vi "GUI.vi"(8 "Error In":errorcluster, 11 "Data in":T6={"Console log"="", "GUI_Events"={"To_GUI-Producer"=refnum, "To_GUI-Error_message"=refnum, "To_GUI-msg_list"=refnum, "To_GUI-Session"=refnum, "To_GUI-Pre-Session"=refnum, "To_GUI-Consumer"=refnum}, "Function_Queue"={"Queue_MIDI_Handler"=refnum, "Queue_Session"=refnum, "Queue_Producer"=refnum, "Queue_Consumer"=refnum}, "Timout-Time[ms]"=0, "MIDI-Messages"=[], "Com Session State"=enum."Active Session", "Result Data"={"Diff"=[], "Tx Byte"=[], "Rx Byte"=[], "Send Log"=[], "Parsed Data"={"Tx MIDI Tag"=[], "Tx MIDI Parsed Data"=[], "Tx Error"=[], "Tx Running States"=[], "Rx MIDI Tag"=[], "Rx MIDI Parsed Data"=[], "Rx Error"=[], "Rx Running States"=[], "Diff"=[]}}, "Get #"=[], "CPU(ms)"=0}) -> (0 "Error Out":errorcluster, 3 "Data out":T6={"Console log"="", "GUI_Events"={"To_GUI-Producer"=refnum, "To_GUI-Error_message"=refnum, "To_GUI-msg_list"=refnum, "To_GUI-Session"=refnum, "To_GUI-Pre-Session"=refnum, "To_GUI-Consumer"=refnum}, "Function_Queue"={"Queue_MIDI_Handler"=refnum, "Queue_Session"=refnum, "Queue_Producer"=refnum, "Queue_Consumer"=refnum}, "Timout-Time[ms]"=0, "MIDI-Messages"=[], "Com Session State"=enum."Active Session", "Result Data"={"Diff"=[], "Tx Byte"=[], "Rx Byte"=[], "Send Log"=[], "Parsed Data"={"Tx MIDI Tag"=[], "Tx MIDI Parsed Data"=[], "Tx Error"=[], "Tx Running States"=[], "Rx MIDI Tag"=[], "Rx MIDI Parsed Data"=[], "Rx Error"=[], "Rx Running States"=[], "Diff"=[]}}, "Get #"=[], "CPU(ms)"=0})   [LabVIEW 2019]
doc: "The main Graphical User Interface"
uses:
  Common/Controls/Application_Data.ctl
  Common/Controls/App_Events.ctl
  Common/Controls/App_Queues.ctl
  Common/Controls/Application_Message.ctl
  Common/Controls/Application_State.ctl
  MIDI/Controls/MIDI-Message_Array.ctl
  MIDI/Controls/MIDI-Message_Cluster.ctl
  MIDI/Controls/Meta_Commands.ctl
  Producer/Controls/Session_State.ctl
  Consumer/Controls/Consumer_Result.ctl
  Consumer/Controls/Parsed_Data.ctl
  Common/Controls/Communication_Protocols.ctl
  Producer/Controls/Serial Settings (Remove).ctl
  <vilib>/Utility/error.llb/DialogType.ctl
  <vilib>/Utility/miscctls.llb/LVPointTypeDef.ctl
  Common/Controls/Communication_Settings.ctl
  Producer/Controls/Prod - Tx_Info.ctl
  <vilib>/Utility/file.llb/Write Delimited Spreadsheet (string).vi
panel:
  in  "BtnG: Minimize":bool
  in  "BtnG: Stop Button":bool
  in  "GUI Tab":T1(tab)
  in  "BtnM: All":bool
  in  "Rx Protocol":T2
  in  "Tx Protocol":T2
  in  "BtnM: Import Send":bool
  in  "BtnM: Preview":bool
  in  "BtnMS: Compose Message":bool
  in  "BtnM: Clear Send":bool
  in  "List: Send":i32(listbox)
  in  "List: MIDI Messages":i32(listbox)
  in  "BtnM: Load Messages":bool
  in  "BtnM: Add to Send":bool
  in  "BtnM: Save":bool
  in  "Custom Message":T3
  in  "BtnM: Cancel/Deinitiate":bool
  in  "BtnM: Initiate Producer":bool
  in  "BtnM: Update Settings":bool
  in  "Serial Communication":T4={"Baud rate"=31250, "Tx Port"="", "Rx Port"=""}
  out "Total amount of bytes to send":i32
  out "Strings":string[](array[string])
  out "Bytesize":i32[](array[numeric])
  out "Datatype":T5[](array[typedef])
  in  "BtnS: Stop Session":bool
  in  "BtnSI: Inspect Session":bool
  in  "BtnS: Pause Session":bool
  in  "BtnS: Start/Resume Session":bool
  in  "BtnI: Inspect Parsing":bool
  out "Diff bytes":i16
  out "Bytes lost":i32
  out "Data error?":bool
  out "Get #":i32
  in  "Get #":bool[](array[boolean])
  in  "BtnI: Save Data as Textfile":bool
  in  "BtnI: Export Send":bool
  in  "Scrollbar":i32(c297)
  out "Send Log":string[](array[string])
  out "Diff":bool[](array[boolean])
  out "Rx Log":string[](array[string])
  out "Tx Log":string[](array[string])
  in  "BtnI: Back 2 Main":bool
  in  "First Rx Failure":i32
  in  "BtnI:  Add Space":bool
  in  "Where Rx should be":i32
  in  "Scrollbar Parse":i32(c297)
  out "Rx Running States":string[](array[string])
  out "Rx Error?":bool[](array[boolean])
  out "Rx MIDI Message Type":string[](array[string])
  out "Rx Parsed Data":string[](array[string])
  out "Diff":bool[](array[boolean])
  out "Tx Error?":bool[](array[boolean])
  out "Tx Running States":string[](array[string])
  out "Tx Parsed Data":string[](array[string])
  out "Tx MIDI Message Type":string[](array[string])
  in  "BtnI: Back 2 Main 2":bool
  out "GUI Console log":string
  out "Error Message":string
  out "Error Loop":string
  out "VI Path":path
  out "VI-filename":string
  out "Revision Number":u32
  out "VI-Name":string
  # "Functions\nDelay:100\nWaitrx\nPause\nLoop"
  # "Important\nAvoid duplicate names"
  # "To Transmit"
  # "Initial Information"
  # "Data loss"
  # "Adds space, in Rx col, where Tx has no corresponding Rx value."
  # "Send-list could be better done:\nBuffer in parallell with send-list, reduces risk of not finding data."
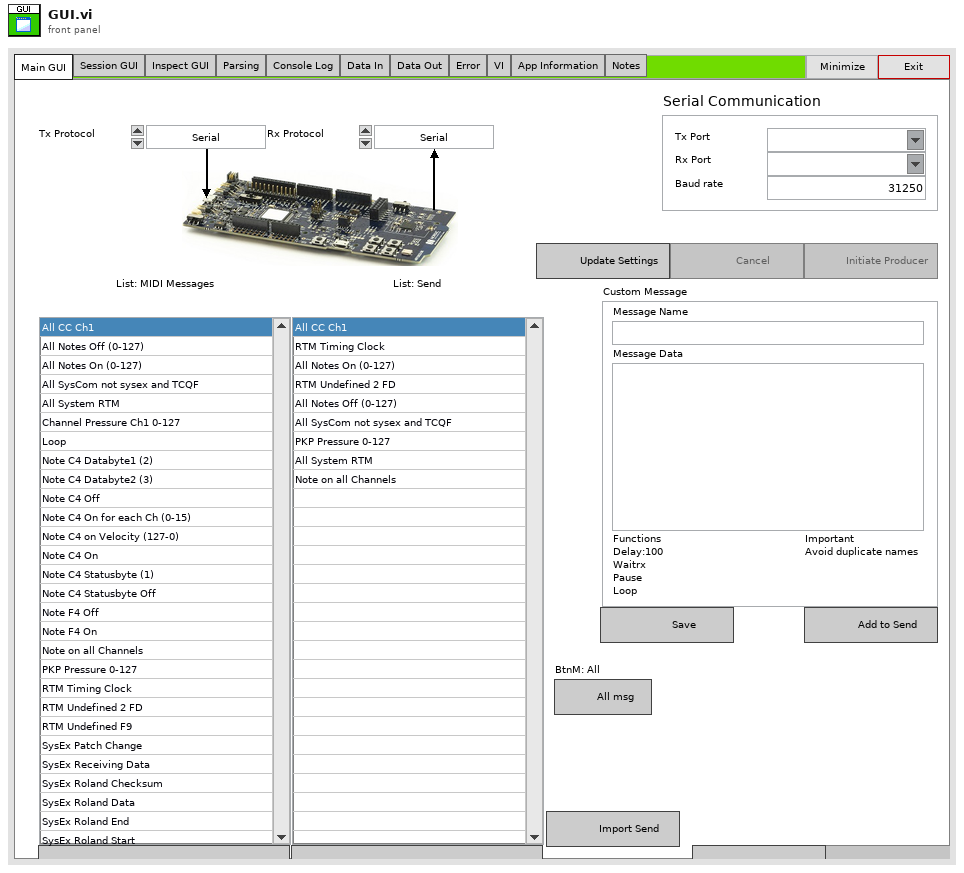
[diagram p1: front panel]
types:
  T1 = enum32{"Main GUI", "Session GUI", "Inspect GUI", "Parsing", "Console Log", "Data In", "Data Out", "Error", "VI", "App Information", "Notes"}
  T2 = typedef "Communication_Protocols.ctl" = enum16{"Serial", "Bluetooth", "USB-MIDI", "MIDI (Audio Device)", "Not Active"}
  T3 = cluster{"Message Name":string, "Message Data":string}
  T4 = typedef "Serial Settings (Remove).ctl" = cluster{"Baud rate":i32, "Tx Port":refnum<visa-resource-name>, "Rx Port":refnum<visa-resource-name>}
  T5 = typedef "Meta_Commands.ctl" = enum16{"No Data", "Pause", "Loop", "Wait for Rx", "Delay", "Break", "MIDI"}
  T6 = typedef "Application_Data.ctl" = cluster{"Console log":string, "GUI_Events":T7, "Function_Queue":T8, "Timout-Time[ms]":i32, "MIDI-Messages":T9, "Com Session State":T11, "Result Data":T12, "Get #":bool[], "CPU(ms)":u32}
  T7 = typedef "App_Events.ctl" = cluster{"To_GUI-Producer":refnum<user-event>, "To_GUI-Error_message":refnum<user-event>, "To_GUI-msg_list":refnum<user-event>, "To_GUI-Session":refnum<user-event>, "To_GUI-Pre-Session":refnum<user-event>, "To_GUI-Consumer":refnum<user-event>}
  T8 = typedef "App_Queues.ctl" = cluster{"Queue_MIDI_Handler":refnum<queue>, "Queue_Session":refnum<queue>, "Queue_Producer":refnum<queue>, "Queue_Consumer":refnum<queue>}
  T9 = typedef "MIDI-Message_Array.ctl" = T10[]
  T10 = typedef "MIDI-Message_Cluster.ctl" = cluster{"Message Name":string, "Meta value":i32, "Datastring":string, "Datatype":T5}
  T11 = typedef "Session_State.ctl" = enum16{"Wait to begin", "Active Session", "Pause", "Wait for Response", "Stop", "Restart", "Inspect", "Exit"}
  T12 = typedef "Consumer_Result.ctl" = cluster{"Diff":bool[], "Tx Byte":string[], "Rx Byte":string[], "Send Log":string[], "Parsed Data":T13}
  T13 = typedef "Parsed_Data.ctl" = cluster{"Tx MIDI Tag":string[], "Tx MIDI Parsed Data":string[], "Tx Error":bool[], "Tx Running States":string[], "Rx MIDI Tag":string[], "Rx MIDI Parsed Data":string[], "Rx Error":bool[], "Rx Running States":string[], "Diff":bool[]}
  T14 = typedef "LVPointTypeDef.ctl" = cluster{"Horizontal":i16, "Vertical":i16}
  T15 = typedef "DialogType.ctl" = u16
  T16 = enum32{"Invalid", "Standard", "Closed", "Hidden", "Minimized", "Maximized"}
  T17 = enum8{"Enabled", "Disabled", "Disabled and Grayed Out"}
  T18 = typedef "Application_Message.ctl" = cluster{"Application State":T19, "Payload":variant}
  T19 = typedef "Application_State.ctl" = enum16{"Idle", "Initiate", "MH Load Messages", "Prepare for Tx", "Settings", "Com Session", "Receive", "Data", "Uninitialize", "Quit Message", "Export Send"}
  T20 = enum16{"open", "replace", "create", "open or create", "replace or create", "replace or create with confirmation"}
  T21 = enum16{"None", "XON/XOFF", "RTS/CTS", "XON/XOFF & RTS/CTS", "DTR/DSR", "XON/XOFF & DTR/DSR"}
  T22 = typedef "Prod - Tx_Info.ctl" = cluster{"Datatype":T5[], "Bytesize":i32[], "Strings":string[], "ByteSum":i32}
  T23 = typedef "Communication_Settings.ctl" = cluster{"Tx Protocol":T2, "Rx Protocol":T2, "Serial":cluster{"Tx Port":refnum<visa-resource-name>, "Rx Port":refnum<visa-resource-name>, "Baud rate":i32, "Parity":enum16{"None", "Odd", "Even", "Mark", "Space"}, "Data bits":i32, "Stop bits":i32, "Flow control":enum16{"None", "XON/XOFF", "RTS/CTS", "XON/XOFF & RTS/CTS", "DTR/DSR", "XON/XOFF & DTR/DSR"}, "Tx Resource":refnum<visa-resource-name>, "Rx Resource":refnum<visa-resource-name>}, "MIDI Device":cluster{"Input uDevice ID":u32, "Output uDevice ID":u32, "hmidiout Handle":i32, "hmidiin Handle":i32}, "Bluetooth":cluster{"Dummy":string}, "USB":cluster{"Dummy":string}}
  T24 = typedef "LVRectTypeDef.ctl" = cluster{"Left":i16, "Top":i16, "Right":i16, "Bottom":i16}
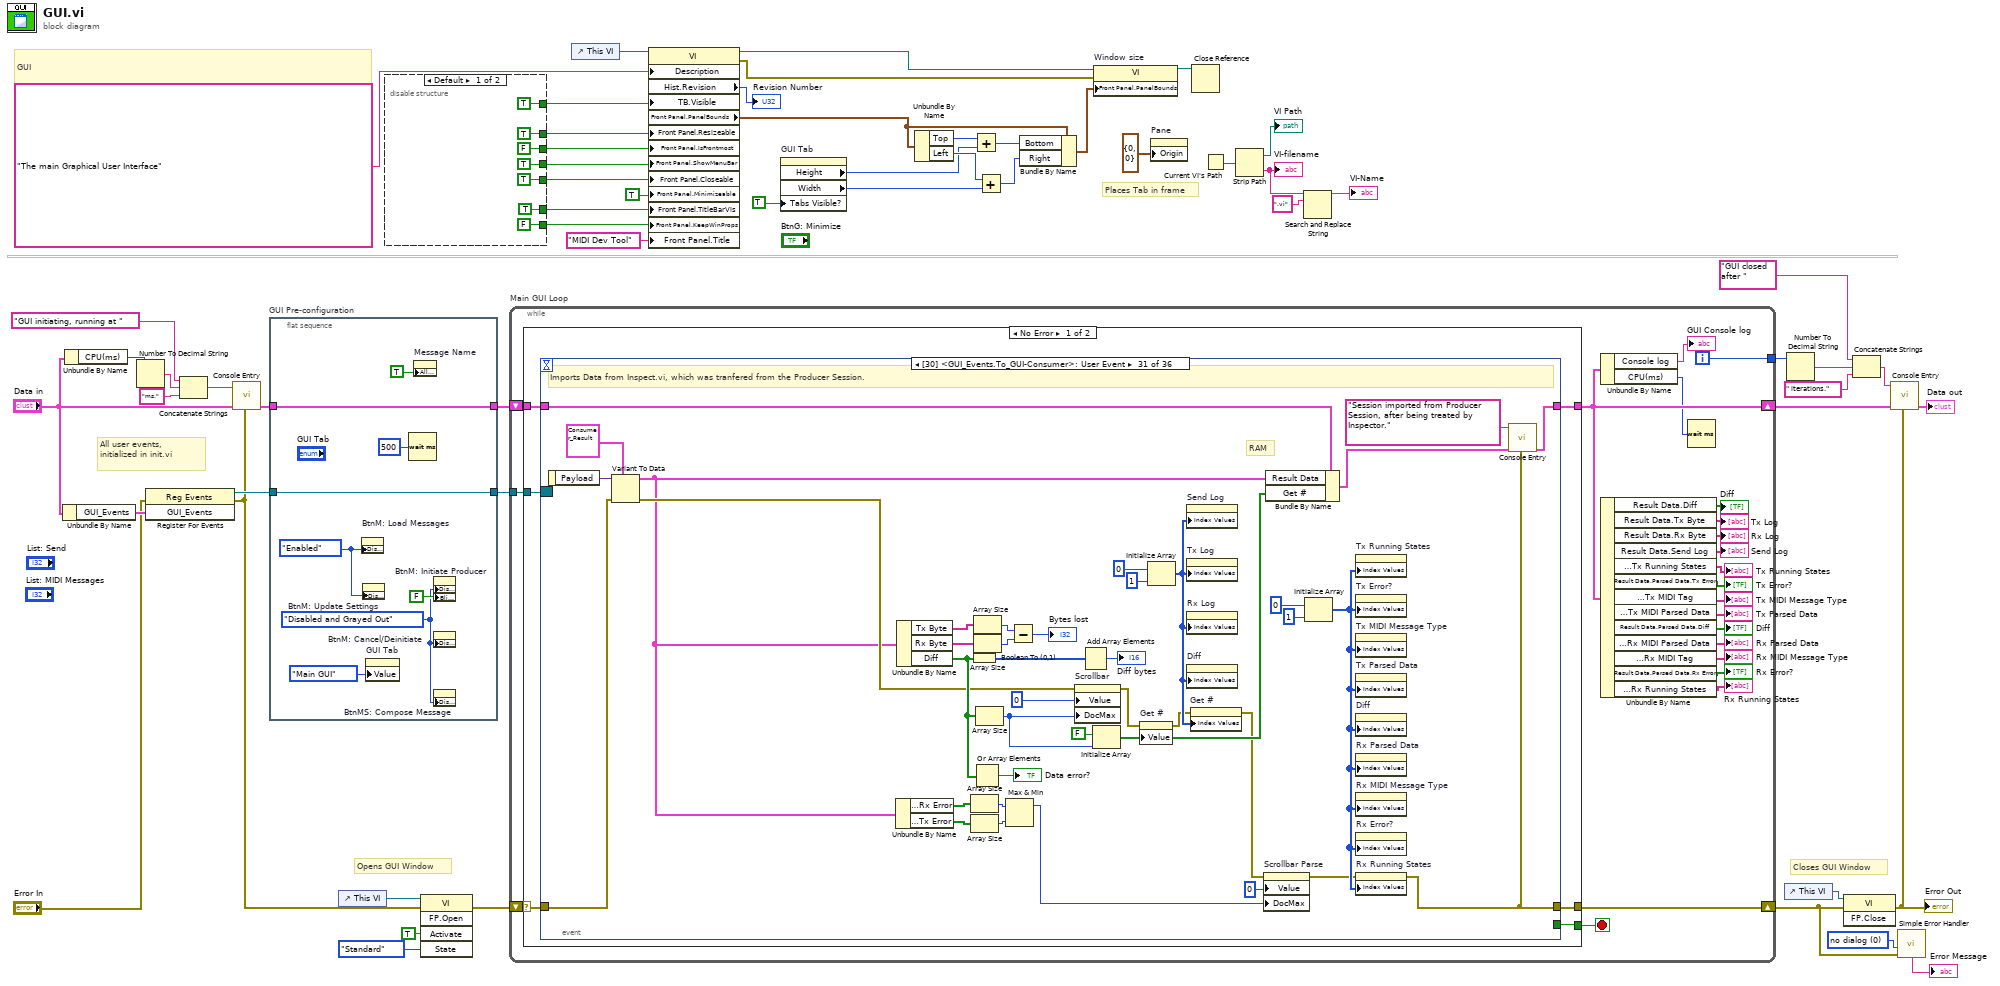
[diagram p0: block diagram]
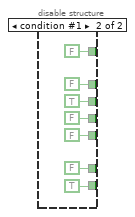
[diagram p2: hidden frame]
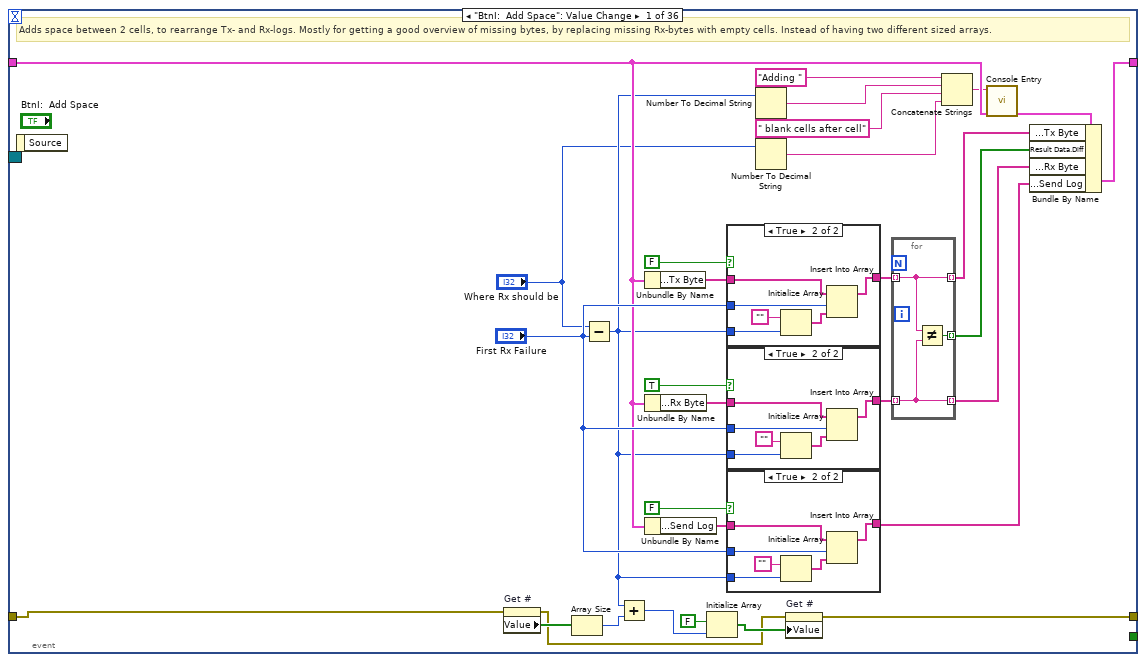
[diagram p3: hidden frame]
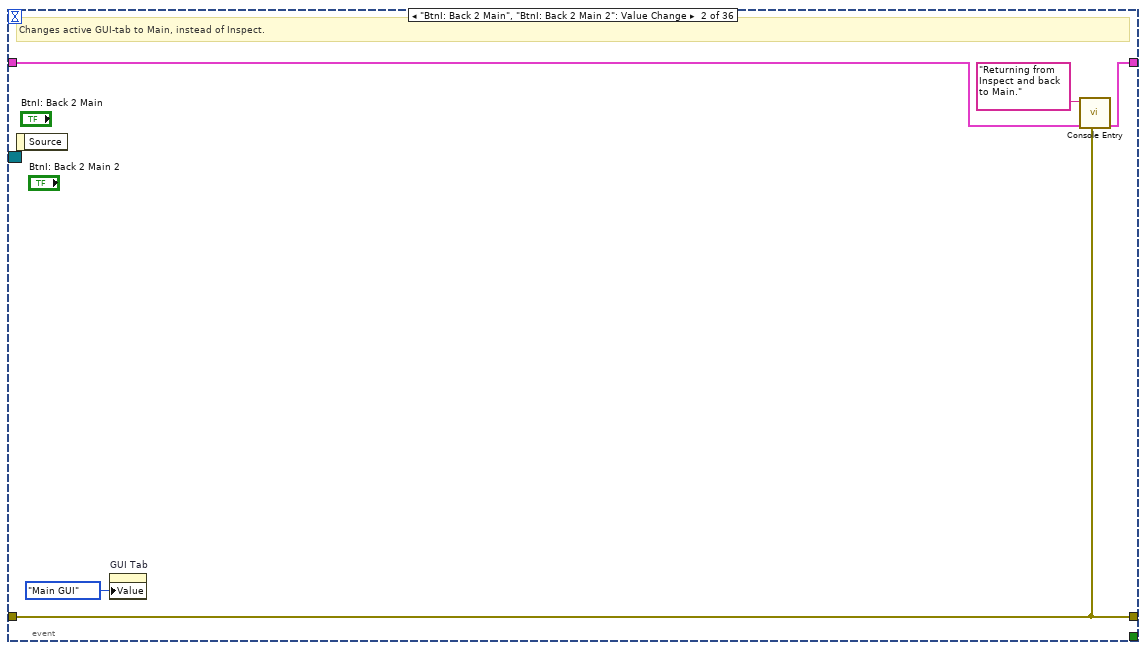
[diagram p7: hidden frame]
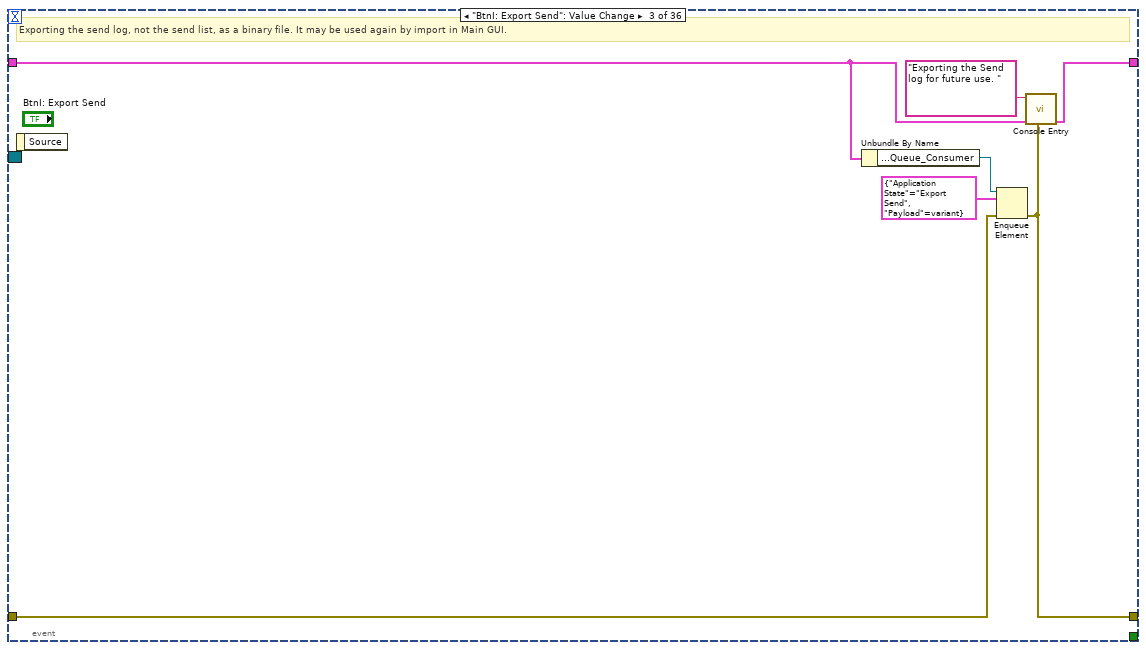
[diagram p8: hidden frame]
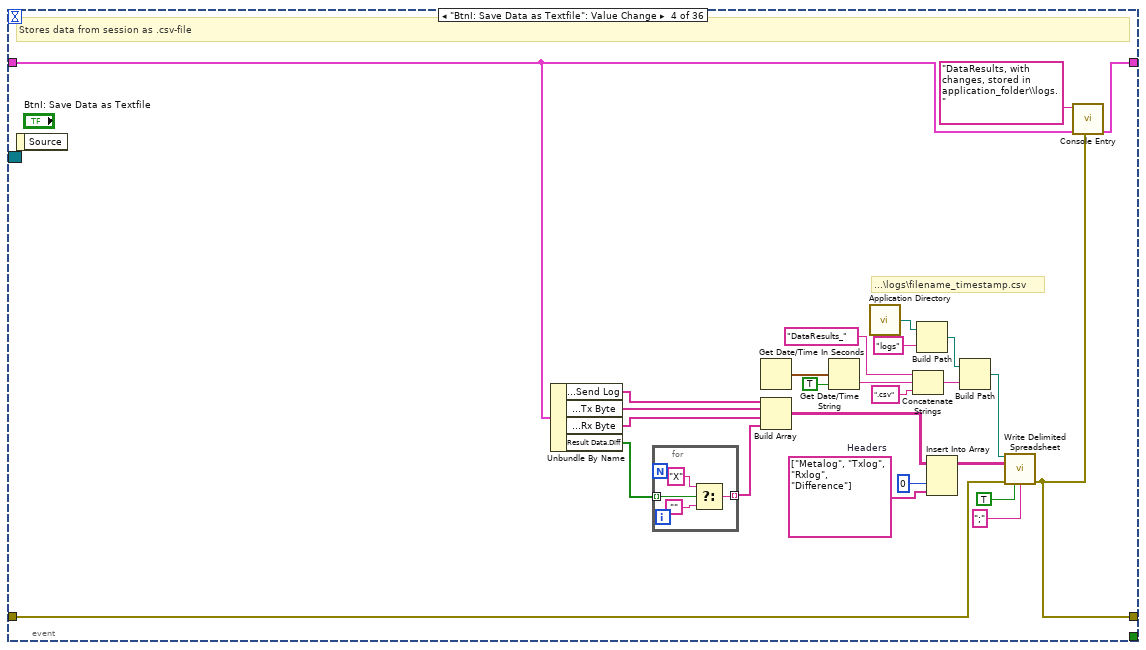
[diagram p9: hidden frame]
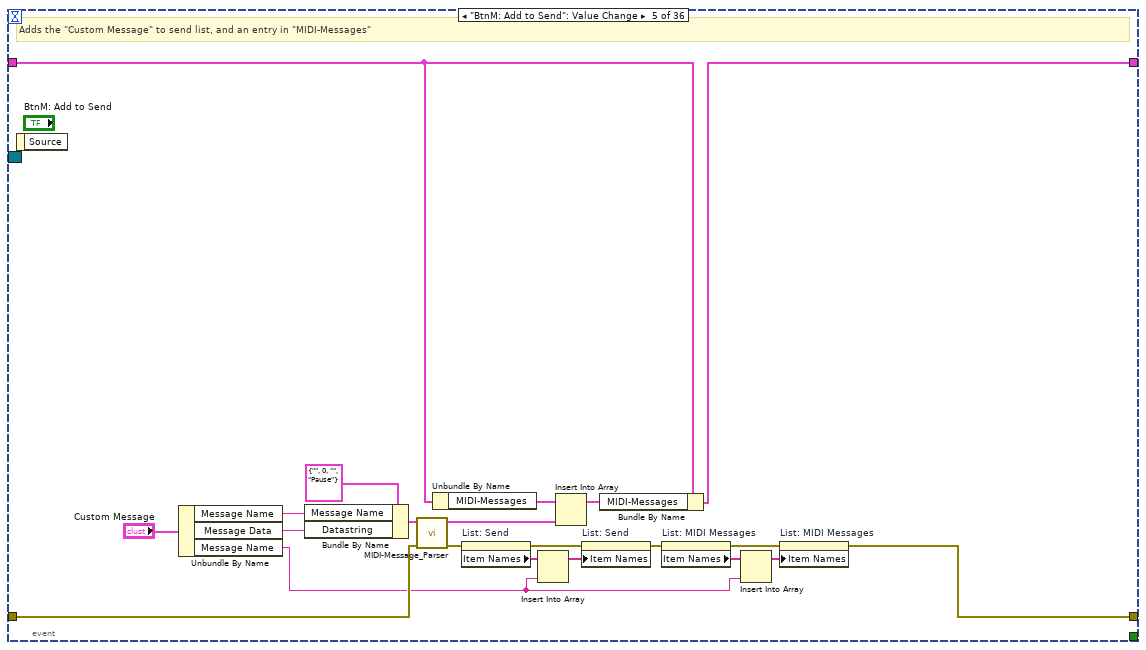
[diagram p10: hidden frame]
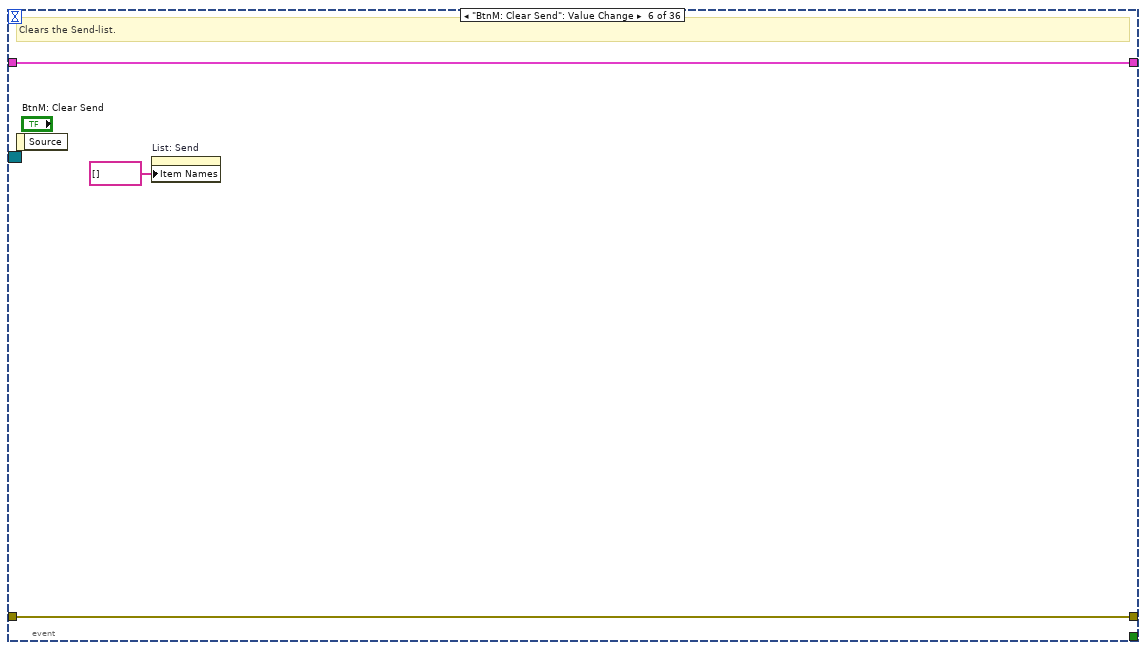
[diagram p11: hidden frame]
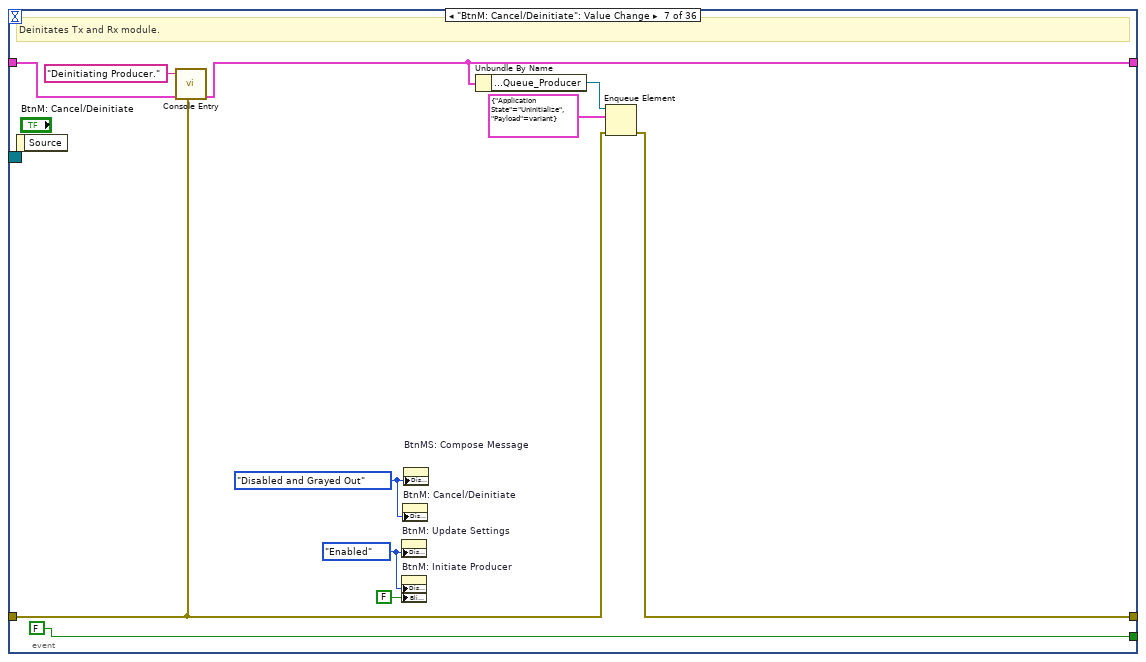
[diagram p12: hidden frame]
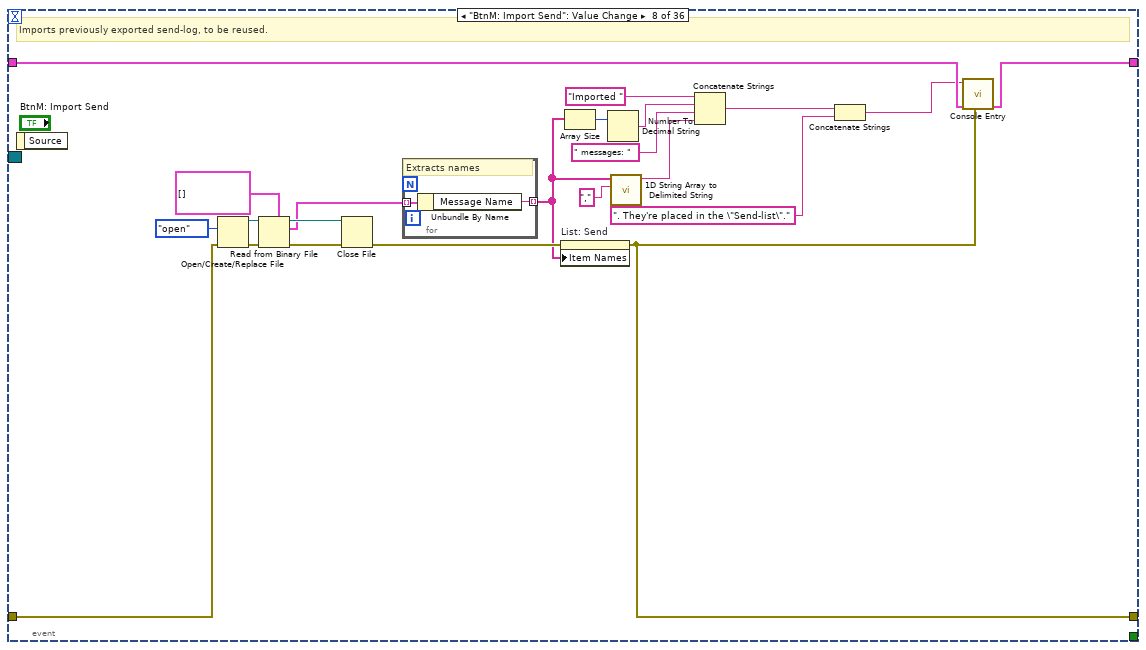
[diagram p13: hidden frame]
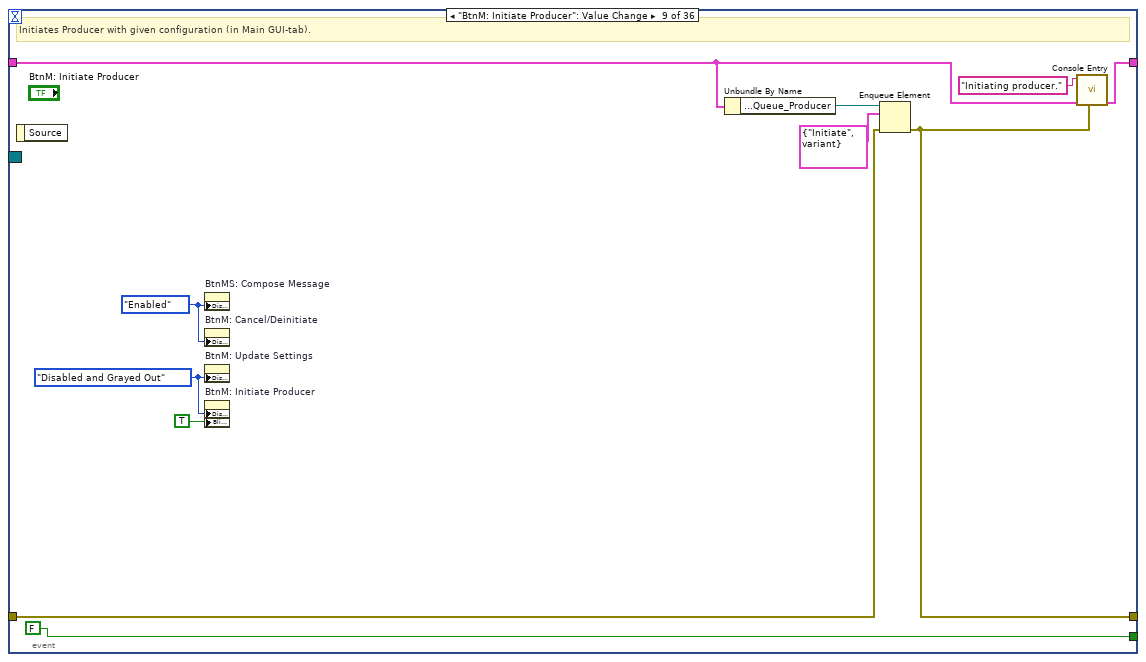
[diagram p14: hidden frame]
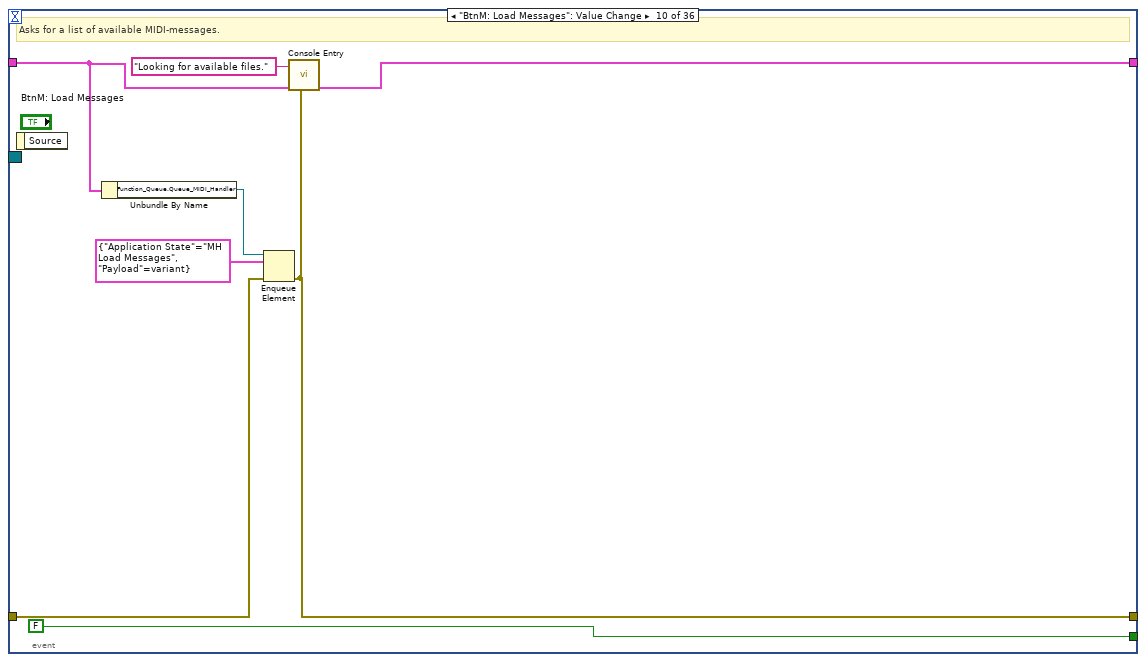
[diagram p15: hidden frame]
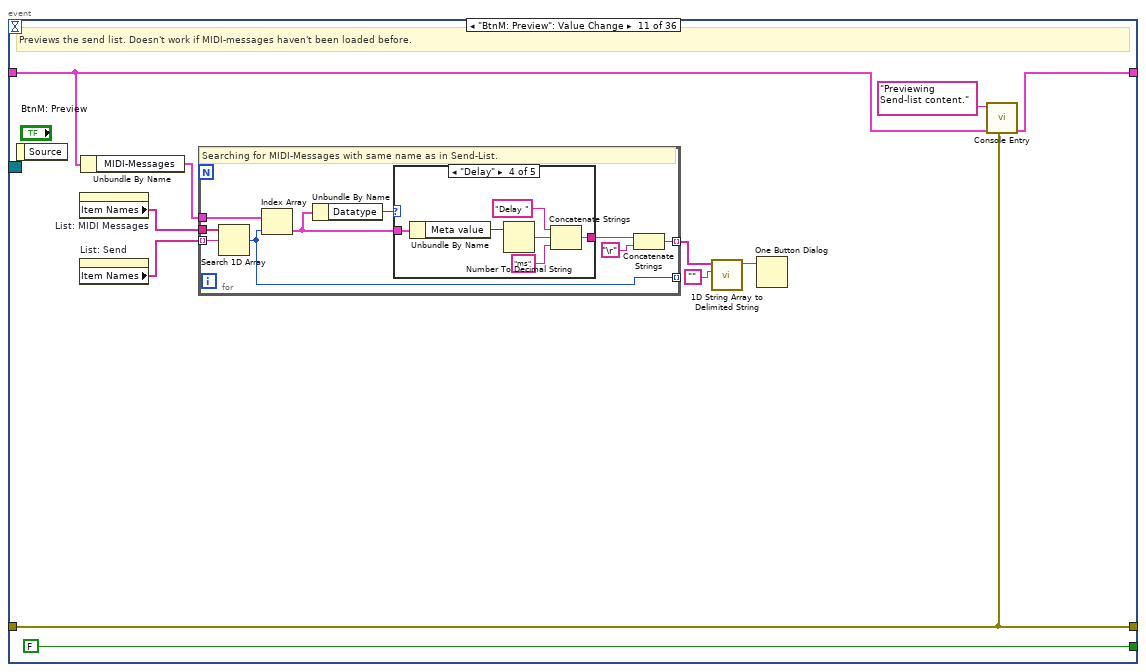
[diagram p16: hidden frame]
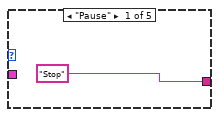
[diagram p17: hidden frame]
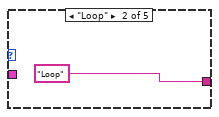
[diagram p18: hidden frame]
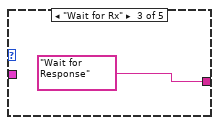
[diagram p19: hidden frame]
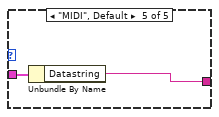
[diagram p20: hidden frame]
diagram:
  w40 = T15 0 items=["no dialog", "OK message", "continue or stop message", "OK message + warnings", "continue/stop + warnings"] ("type of dialog (OK msg:1)")
  # "Places Tab in frame"
  # "GUI"
  # "All user events, initialized in init.vi"
  # "Closes GUI Window"
  # "Opens GUI Window"
  n1 = Unbundle By Name("Data in") -> ("GUI_Events"=w49:T7)
  n2 = Unbundle By Name("Data in") -> ("CPU(ms)"=w34:u32)
  n3 = Number To Decimal String(number=w34) -> (decimal integer string=w31:string)  [unwired: 1 in]
  n4 = register-events(error in="Error In", w49) -> (reference out=w51:refnum<event-registration>, error out=w29:errorcluster)  [unwired: 1 in]
  n5 = Concatenate Strings("GUI initiating, running at " ("Console Entry"), w31, "ms." ("string")) -> (w33:string)
  n6 = call "Console Entry.vi"("Error In"=w29, "Data In"="Data in", "Console Entry"=w33) -> ("Data out"=w44:T6)  [unwired: 8 in]
  n7 = flat-sequence "GUI Pre-configuration" {
    tunnel: w44 -> [w67]
    tunnel: [w67] -> w52
    tunnel: w51 -> [w66]
    tunnel: [w66] -> w50
    frame #0 {
      w63 = T17."Enabled" ("Disabled")
      w62 = T17."Disabled and Grayed Out" ("Disabled")
      n8 = property on="BtnM: Load Messages" class="Bool"("DisabledEnum"=w63) -> ()  [unwired: 2 in, 2 out]
      n9 = property on="BtnM: Update Settings" class="Bool"("DisabledEnum"=w63) -> ()  [unwired: 2 in, 2 out]
      n10 = property on="GUI Tab" class="TabCtl (strict)"("Value"=T1."Main GUI" ("GUI Tab")) -> ()  [unwired: 2 in, 2 out]
      n11 = Wait (ms)(milliseconds to wait=u32 500) -> ()  [unwired: 1 out]
      n12 = property on="Message Name" class="Str"("AllowDrop"=TRUE ("Allow Dropping")) -> ()  [unwired: 2 in, 2 out]
      n13 = property on="BtnM: Initiate Producer" class="Bool"("DisabledEnum"=w62, "Blinking"=FALSE) -> ()  [unwired: 2 in, 2 out]
      n14 = property on="BtnM: Cancel/Deinitiate" class="Bool"("DisabledEnum"=w62) -> ()  [unwired: 2 in, 2 out]
      n15 = property on="BtnMS: Compose Message" class="Bool"("DisabledEnum"=w62) -> ()  [unwired: 2 in, 2 out]
    }
  }
  n16 = control-ref of="This VI"() -> (w57:refnum<vi>)
  n17 = disable-structure "Exe vs Sim" shown="Default" {
    disable-tunnel: [TRUE ("Tool Bar:Visible") FALSE ("Tool Bar:Visible")] -> w9
    disable-tunnel: [FALSE ("Front Panel Window:Is Frontmost") TRUE ("Front Panel Window:Is Frontmost")] -> w8
    disable-tunnel: [TRUE ("Front Panel Window:Show Menu Bar") FALSE ("Front Panel Window:Show Menu Bar")] -> w7
    disable-tunnel: [TRUE ("Front Panel Window:Resizable") FALSE ("Front Panel Window:Resizable")] -> w6
    disable-tunnel: [TRUE ("Front Panel Window:Closeable") FALSE ("Front Panel Window:Closeable")] -> w4
    disable-tunnel: [TRUE ("Front Panel Window:Title Bar Visible") FALSE ("Front Panel Window:Title Bar Visible")] -> w3
    disable-tunnel: [FALSE ("Front Panel Window:Title Bar Visible") TRUE ("Front Panel Window:Title Bar Visible")] -> w1
    frame condition #0 (active) {
    }
    frame condition #1 {
    }
  }
  n18 = invoke on="Invoke Node" class="VI" method="FP.Open"(reference=w57, error in=w29, "Activate"=TRUE ("Activate?"), "State"=T16."Standard") -> (error out=w54:errorcluster)  [unwired: 1 in, 4 out]
  n19 = while "Main GUI Loop" {
    shift-right: [w102] -> w41
    shift-left: w54 -> [w103]
    shift-right: [w97] -> w43
    shift-left: w52 -> [w100]
    tunnel: w50 -> [w99]
    tunnel: [w91] -> w25
    i -> [w91]
    stop <- w101 stop-if-true
    n20 = case shown="No Error" w103 {
      selector: w103 -> [w105 w839]
      tunnel: [w109 w839] -> w102
      tunnel: [w106 w843] -> w101
      tunnel: w100 -> [w108 w841]
      tunnel: [w104 w842] -> w97
      tunnel: w99 -> [w107 _]
      frame No Error {
        n21 = event shown="[30] <GUI_Events.To_GUI-Consumer>: User Event" {
          selector: w107 -> [_ _ _ _ _ _ _ _ _ _ _ _ _ _ _ _ _ _ _ _ _ _ _ _ _ _ _ _ _ _ _ _ _ _ _ _]
          dyn-events: _ -> [_ _ _ _ _ _ _ _ _ _ _ _ _ _ _ _ _ _ _ _ _ _ _ _ _ _ _ _ _ _ _ _ _ _ _ _]
          timeout: _ -> [_ _ _ _ _ _ _ _ _ _ _ _ _ _ _ _ _ _ _ _ _ _ _ _ _ _ _ _ _ _ _ _ _ _ _ _]
          tunnel: [w127 w166 w171 w177 w216 w228 w233 w245 w270 w278 w286 w319 w352 w370 w388 w393 w417 w454 w500 w544 w568 w599 w631 w639 w644 w656 w672 w689 w701 w716 w731 w761 w774 w788 w799 w838] -> w109
          tunnel: w105 -> [w129 w166 w174 w201 w210 w228 w231 w263 w271 w279 w286 w328 w353 w371 w391 w394 w418 w469 w519 w548 w561 w596 w632 w640 w647 w661 w680 w696 w707 w717 w759 w769 w782 w795 w804 w838]
          tunnel: w108 -> [w118 w168 w172 w178 w225 w230 w236 w247 w266 w281 w287 w330 w355 w373 w392 w396 w420 w458 w502 w550 w563 w598 w634 w642 w646 w658 w674 w690 w703 w719 w753 w763 w779 w787 w803 w836]
          tunnel: [_ _ _ _ _ _ FALSE ("Shutdown Program") _ FALSE ("Shutdown Program") FALSE ("Shutdown Program") FALSE ("Shutdown Program") _ TRUE ("Shutdown Program") TRUE ("Shutdown Program") _ TRUE ("Shutdown Program") FALSE ("Shutdown Program") _ FALSE ("Shutdown Program") _ _ _ _ _ _ _ FALSE ("Shutdown Program") _ _ _ _ FALSE ("Shutdown Program") _ _ _ FALSE ("Shutdown Program")] -> w106
          tunnel: [w135 w167 w173 w180 w226 w230 w232 w246 w269 w282 w288 w317 w354 w372 w392 w395 w419 w473 w503 w545 w569 w592 w630 w642 w645 w659 w673 w687 w702 w719 w736 w762 w775 w789 w801 w836] -> w104
          event "BtnI:  Add Space": Value Change {
            # "Adds space between 2 cells, to rearrange Tx- and Rx-logs. Mostly for getting a good overview of missing bytes, by replacing missing Rx-bytes with empty cells. Instead of having two different sized arrays."
            n22 = event-data() -> ()  [unwired: 1 in, 1 out]
            n23 = property on="Get #" class="Arr (strict)"(error in=w129) -> (error out=w128:errorcluster, "Value"=w134:bool[])  [unwired: 1 in, 1 out]
            n24 = Array Size(array=w134) -> (size(s)=w132:i32)
            n25 = Subtract(x="Where Rx should be", y="First Rx Failure") -> (x-y=w111:i32)
            n26 = Add(x=w111, y=w132) -> (x+y=w133:i32)
            n27 = Unbundle By Name(w118) -> ("Result Data.Tx Byte"=w140:string[])
            n28 = Unbundle By Name(w118) -> ("Result Data.Rx Byte"=w139:string[])
            n29 = Unbundle By Name(w118) -> ("Result Data.Send Log"=w138:string[])
            n30 = Initialize Array(FALSE, w133) -> (w130:bool[])
            n31 = case shown="True" FALSE ("Insertspace: Tx 2") {
              tunnel: w140 -> [w158 w164]
              tunnel: [w158 w163] -> w124
              tunnel: "First Rx Failure" -> [_ w162]
              tunnel: w111 -> [_ w161]
              frame False {
              }
              frame True {
                n32 = Initialize Array("", w161) -> (w160:string[])
                n33 = Insert Into Array(array=w164, index=w162, new element=w160) -> (w163:string[])
              }
            }
            n34 = case shown="True" TRUE ("Insertspace: Rx 2") {
              tunnel: w139 -> [w151 w157]
              tunnel: [w151 w156] -> w123
              tunnel: "First Rx Failure" -> [_ w155]
              tunnel: w111 -> [_ w154]
              frame False {
              }
              frame True {
                n35 = Initialize Array("", w154) -> (w153:string[])
                n36 = Insert Into Array(array=w157, index=w155, new element=w153) -> (w156:string[])
              }
            }
            n37 = case shown="True" FALSE ("Insertspace:\nSend 2") {
              tunnel: w138 -> [w144 w150]
              tunnel: [w144 w149] -> w136
              tunnel: "First Rx Failure" -> [_ w148]
              tunnel: w111 -> [_ w147]
              frame False {
              }
              frame True {
                n38 = Initialize Array("", w147) -> (w146:string[])
                n39 = Insert Into Array(array=w150, index=w148, new element=w146) -> (w149:string[])
              }
            }
            n40 = Number To Decimal String(number=w111) -> (decimal integer string=w115:string)  [unwired: 1 in]
            n41 = Number To Decimal String(number="Where Rx should be") -> (decimal integer string=w112:string)  [unwired: 1 in]
            n42 = property on="Get #" class="Arr (strict)"(error in=w128, "Value"=w130) -> (error out=w127:errorcluster)  [unwired: 1 in, 1 out]
            n43 = for {
              tunnel: w124 -> [w142] mode=indexing
              tunnel: w123 -> [w141] mode=indexing
              tunnel: [w143] -> w120 mode=indexing
              tunnel: [w142] -> w121 mode=indexing
              tunnel: [w141] -> w122 mode=indexing
              n44 = Not Equal?(x=w142, y=w141) -> (x != y?=w143:bool)
            }
            n45 = Concatenate Strings("Adding ", w115, " blank cells after cell" ("string"), w112) -> (w113:string)
            n46 = call "Console Entry.vi"("Data In"=w118, "Console Entry"=w113) -> ("Data out"=w117:T6)  [unwired: 9 in]
            n47 = Bundle By Name(cluster=w117, "Result Data.Tx Byte"=w121, "Result Data.Diff"=w120, "Result Data.Rx Byte"=w122, "Result Data.Send Log"=w136) -> (w135:T6)
          }
          event "BtnI: Back 2 Main", "BtnI: Back 2 Main 2": Value Change {
            # "Changes active GUI-tab to Main, instead of Inspect."
            n48 = event-data() -> ()  [unwired: 1 in, 1 out]
            n49 = property on="GUI Tab" class="TabCtl (strict)"("Value"=T1."Main GUI" ("GUI Tab")) -> ()  [unwired: 2 in, 2 out]
            n50 = call "Console Entry.vi"("Error In"=w166, "Data In"=w168, "Console Entry"="Returning from Inspect and back to Main.") -> ("Data out"=w167:T6)  [unwired: 8 in]
          }
          event "BtnI: Export Send": Value Change {
            # "Exporting the send log, not the send list, as a binary file. It may be used again by import in Main GUI."
            n51 = event-data() -> ()  [unwired: 1 in, 1 out]
            n52 = Unbundle By Name(w172) -> ("Function_Queue.Queue_Consumer"=w176:refnum<queue>)
            n53 = Enqueue Element(queue=w176, element=T18 {"Application State"=enum."Export Send", "Payload"=variant}, error in (no error)=w174) -> (error out=w171:errorcluster)  [unwired: 1 in, 2 out]
            n54 = call "Console Entry.vi"("Error In"=w171, "Data In"=w172, "Console Entry"="Exporting the Send log for future use. ") -> ("Data out"=w173:T6)  [unwired: 8 in]
          }
          event "BtnI: Save Data as Textfile": Value Change {
            w186 = string[] ["Metalog", "Txlog", "Rxlog", "Difference"]  # Headers
            # "...\\logs\\filename_timestamp.csv"
            # "Stores data from session as .csv-file"
            n55 = event-data() -> ()  [unwired: 1 in, 1 out]
            n56 = Unbundle By Name(w178) -> ("Result Data.Send Log"=w191:string[], "Result Data.Tx Byte"=w190:string[], "Result Data.Rx Byte"=w189:string[], "Result Data.Diff"=w202:bool[])
            n57 = for {
              tunnel: w202 -> [w206] mode=indexing
              tunnel: [w203] -> w188 mode=indexing
              n58 = Select(t="X", s=w206, f="") -> (s? t:f=w203:string)
            }
            n59 = Get Date/Time In Seconds() -> (seconds since 1Jan1904=w194:timestamp)
            n60 = Build Array(w191, w190, w189, w188) -> (w187:string[][])
            n61 = Get Date/Time String(seconds (now)=w194, want seconds? (F)=TRUE) -> (time string=w193:string)  [unwired: 1 in, 1 out]
            n62 = call <vilib>:"Application Directory.vi"() -> ("Application Directory"=w181:path)
            n63 = Concatenate Strings("DataResults_" ("string"), w193, ".csv" ("string")) -> (w197:string)
            n64 = Build Path(base path=w181, name or relative path="logs") -> (appended path=w198:path)
            n65 = Insert Into Array(array=w187, index (col)=0 ("index (row)"), new element=w186) -> (w185:string[][])  [unwired: 1 in]
            n66 = Build Path(base path=w198, name or relative path=w197) -> (appended path=w192:path)
            n67 = call-poly <vilib>:"Write Delimited Spreadsheet.vi"("file path (dialog if empty)"=w192, "2D data"=w185, "error in (no error)"=w201, "transpose? (no:F)"=TRUE, "delimiter (\\t)"=";" ("delimiter (\\t)")) -> ("error out"=w177:errorcluster)  [unwired: 9 in, 1 out]
            n68 = call "Console Entry.vi"("Error In"=w177, "Data In"=w178, "Console Entry"="DataResults, with changes, stored in application_folder\\logs.") -> ("Data out"=w180:T6)  [unwired: 8 in]
          }
          event "BtnM: Add to Send": Value Change {
            # "Adds the \"Custom Message\" to send list, and an entry in \"MIDI-Messages\""
            n69 = event-data() -> ()  [unwired: 1 in, 1 out]
            n70 = Unbundle By Name("Custom Message") -> ("Message Name"=w214:string, "Message Data"=w213:string, "Message Name"=w208:string)
            n71 = Bundle By Name(cluster=T10 {"Message Name"="", "Meta value"=0, "Datastring"="", "Datatype"=enum."Pause"} ("MIDI Message Cluster In"), "Message Name"=w214, "Datastring"=w213) -> (w212:T10)
            n72 = call "MIDI-Message_Parser.vi"("Error In"=w210, "MIDI Message Cluster In"=w212) -> ("Error Out"=w209:errorcluster, "MIDI Message Cluster Out"=w211:T10)  [unwired: 8 in]
            n73 = Unbundle By Name(w225) -> ("MIDI-Messages"=w227:T9)
            n74 = property on="List: Send" class="LstBox (strict)"(error in=w209) -> (error out=w217:errorcluster, "Item Names"=w223:string[])  [unwired: 1 in, 1 out]
            n75 = Insert Into Array(array=w223, new element=w208) -> (w222:string[])  [unwired: 1 in]
            n76 = Insert Into Array(array=w227, new element=w211) -> (w224:T9)  [unwired: 1 in]
            n77 = property on="List: Send" class="LstBox (strict)"(error in=w217, "Item Names"=w222) -> (error out=w218:errorcluster)  [unwired: 1 in, 1 out]
            n78 = Bundle By Name(cluster=w225, "MIDI-Messages"=w224) -> (w226:T6)
            n79 = property on="List: MIDI Messages" class="LstBox (strict)"(error in=w218) -> (error out=w219:errorcluster, "Item Names"=w221:string[])  [unwired: 1 in, 1 out]
            n80 = Insert Into Array(array=w221, new element=w208) -> (w220:string[])  [unwired: 1 in]
            n81 = property on="List: MIDI Messages" class="LstBox (strict)"(error in=w219, "Item Names"=w220) -> (error out=w216:errorcluster)  [unwired: 1 in, 1 out]
          }
          event "BtnM: Clear Send": Value Change {
            # "Clears the Send-list."
            n82 = event-data() -> ()  [unwired: 1 in, 1 out]
            n83 = property on="List: Send" class="LstBox (strict)"("Item Names"=string[] []) -> ()  [unwired: 2 in, 2 out]
          }
          event "BtnM: Cancel/Deinitiate": Value Change {
            w234 = T17."Disabled and Grayed Out" ("Disabled")
            w235 = T17."Enabled" ("Disabled")
            # "Deinitates Tx and Rx module."
            n84 = event-data() -> ()  [unwired: 1 in, 1 out]
            n85 = call "Console Entry.vi"("Error In"=w231, "Data In"=w236, "Console Entry"="Deinitiating Producer.") -> ("Data out"=w232:T6)  [unwired: 8 in]
            n86 = property on="BtnM: Update Settings" class="Bool"("DisabledEnum"=w235) -> ()  [unwired: 2 in, 2 out]
            n87 = property on="BtnM: Initiate Producer" class="Bool"("DisabledEnum"=w235, "Blinking"=FALSE) -> ()  [unwired: 2 in, 2 out]
            n88 = property on="BtnM: Cancel/Deinitiate" class="Bool"("DisabledEnum"=w234) -> ()  [unwired: 2 in, 2 out]
            n89 = property on="BtnMS: Compose Message" class="Bool"("DisabledEnum"=w234) -> ()  [unwired: 2 in, 2 out]
            n90 = Unbundle By Name(w232) -> ("Function_Queue.Queue_Producer"=w238:refnum<queue>)
            n91 = Enqueue Element(queue=w238, element=T18 {"Application State"=enum."Uninitialize", "Payload"=variant}, error in (no error)=w231) -> (error out=w233:errorcluster)  [unwired: 1 in, 2 out]
          }
          event "BtnM: Import Send": Value Change {
            # "Imports previously exported send-log, to be reused."
            n92 = event-data() -> ()  [unwired: 1 in, 1 out]
            n93 = Open/Create/Replace File(error in=w263, operation (0:open)=T20."open") -> (refnum out=w260:refnum<file>, error out=w261:errorcluster)  [unwired: 4 in, 1 out]
            n94 = Read from Binary File(5:T9 [] ("MIDI Message Array"), 8:w261, 11:w260) -> (0:w257:errorcluster, 2:w256:T9, 3:w258:refnum<file>)  [unwired: 3 in, 1 out]
            n95 = Close File(refnum=w258, error in=w257) -> (error out=w255:errorcluster)  [unwired: 1 out]
            n96 = for {
              tunnel: w256 -> [w265] mode=indexing
              tunnel: [w264] -> w250 mode=indexing
              # "Extracts names"
              n97 = Unbundle By Name(w265) -> ("Message Name"=w264:string)
            }
            n98 = property on="List: Send" class="LstBox (strict)"(error in=w255, "Item Names"=w250) -> (error out=w245:errorcluster)  [unwired: 1 in, 1 out]
            n99 = Array Size(array=w250) -> (size(s)=w254:i32)
            n100 = Number To Decimal String(number=w254) -> (decimal integer string=w252:string)  [unwired: 1 in]
            n101 = call <vilib>:"1D String Array to Delimited String.vi"("delimiter"=",", "string array"=w250) -> ("delimited string"=w249:string)  [unwired: 9 in]
            n102 = Concatenate Strings("Imported " ("string"), w252, " messages: " ("string"), w249) -> (w244:string)
            n103 = Concatenate Strings(w244, ". They're placed in the \"Send-list\"." ("string")) -> (w243:string)
            n104 = call "Console Entry.vi"("Error In"=w245, "Data In"=w247, "Console Entry"=w243) -> ("Data out"=w246:T6)  [unwired: 8 in]
          }
          event "BtnM: Initiate Producer": Value Change {
            w267 = T17."Enabled" ("Disabled")
            w268 = T17."Disabled and Grayed Out" ("Disabled")
            # "Initiates Producer with given configuration (in Main GUI-tab)."
            n105 = event-data() -> ()  [unwired: 1 in, 1 out]
            n106 = property on="BtnMS: Compose Message" class="Bool"("DisabledEnum"=w267) -> ()  [unwired: 2 in, 2 out]
            n107 = property on="BtnM: Cancel/Deinitiate" class="Bool"("DisabledEnum"=w267) -> ()  [unwired: 2 in, 2 out]
            n108 = property on="BtnM: Update Settings" class="Bool"("DisabledEnum"=w268) -> ()  [unwired: 2 in, 2 out]
            n109 = property on="BtnM: Initiate Producer" class="Bool"("DisabledEnum"=w268, "Blinking"=TRUE) -> ()  [unwired: 2 in, 2 out]
            n110 = Unbundle By Name(w266) -> ("Function_Queue.Queue_Producer"=w273:refnum<queue>)
            n111 = Enqueue Element(queue=w273, element=T18 {"Application State"=enum."Initiate", "Payload"=variant}, error in (no error)=w271) -> (error out=w270:errorcluster)  [unwired: 1 in, 2 out]
            n112 = call "Console Entry.vi"("Error In"=w270, "Data In"=w266, "Console Entry"="Initiating producer.") -> ("Data out"=w269:T6)  [unwired: 8 in]
          }
          event "BtnM: Load Messages": Value Change {
            # "Asks for a list of available MIDI-messages."
            n113 = event-data() -> ()  [unwired: 1 in, 1 out]
            n114 = Unbundle By Name(w281) -> ("Function_Queue.Queue_MIDI_Handler"=w280:refnum<queue>)
            n115 = Enqueue Element(queue=w280, element=T18 {"Application State"=enum."MH Load Messages", "Payload"=variant} ("Application Message"), error in (no error)=w279) -> (error out=w278:errorcluster)  [unwired: 1 in, 2 out]
            n116 = call "Console Entry.vi"("Error In"=w278, "Data In"=w281, "Console Entry"="Looking for available files.") -> ("Data out"=w282:T6)  [unwired: 8 in]
          }
          event "BtnM: Preview": Value Change {
            # "Previews the send list. Doesn't work if MIDI-messages haven't been loaded before."
            n117 = event-data() -> ()  [unwired: 1 in, 1 out]
            n118 = property on="List: MIDI Messages" class="LstBox (strict)"() -> ("Item Names"=w294:string[])  [unwired: 2 in, 2 out]
            n119 = property on="List: Send" class="LstBox (strict)"() -> ("Item Names"=w295:string[])  [unwired: 2 in, 2 out]
            n120 = Unbundle By Name(w287) -> ("MIDI-Messages"=w293:T9)
            n121 = for {
              tunnel: w295 -> [w304] mode=indexing
              tunnel: w294 -> [w303]
              tunnel: w293 -> [w302]
              tunnel: [w301] -> _ mode=indexing
              tunnel: [w296] -> w292 mode=indexing
              # "Searching for MIDI-Messages with same name as in Send-List."
              n122 = Search 1D Array(1D array=w303, element=w304) -> (index of element=w301:i32)  [unwired: 1 in]
              n123 = Index Array(array=w302, index=w301) -> (element=w299:T10)
              n124 = Unbundle By Name(w299) -> ("Datatype"=w300:T5)
              n125 = case shown="\"Delay\"" w300 {
                tunnel: w299 -> [_ _ _ w313 w315]
                tunnel: ["Stop" ("Datastring") "Loop" ("Datastring") "Wait for Response" ("Datastring") w308 w314] -> w298
                frame "Pause" {
                }
                frame "Loop" {
                }
                frame "Wait for Rx" {
                }
                frame "Delay" {
                  n126 = Unbundle By Name(w313) -> ("Meta value"=w312:i32)
                  n127 = Number To Decimal String(number=w312) -> (decimal integer string=w311:string)  [unwired: 1 in]
                  n128 = Concatenate Strings("Delay " ("string"), w311, "ms" ("string")) -> (w308:string)
                }
                frame "MIDI", Default {
                  n129 = Unbundle By Name(w315) -> ("Datastring"=w314:string)
                }
              }
              n130 = Concatenate Strings(w298, "\r") -> (w296:string)
            }
            n131 = call <vilib>:"1D String Array to Delimited String.vi"("delimiter"="", "string array"=w292) -> ("delimited string"=w290:string)  [unwired: 9 in]
            n132 = One Button Dialog(message=w290) -> ()  [unwired: 1 in, 1 out]
            n133 = call "Console Entry.vi"("Error In"=w286, "Data In"=w287, "Console Entry"="Previewing Send-list content.") -> ("Data out"=w288:T6)  [unwired: 8 in]
          }
          event "BtnM: Save": Value Change {
            # "Saves the \"Custom Message\" to the \"midi_message\"-folder. Messages in \"MIDI Messages\" are reloaded. This could be moved to the MIDI-generator."
            n134 = event-data() -> ()  [unwired: 1 in, 1 out]
            n135 = local read "Custom Message"() -> (w335:T3)
            n136 = Unbundle By Name(w335) -> ("Message Name"=w326:string, "Message Data"=w322:string)
            n137 = call <vilib>:"Application Directory.vi"() -> ("Application Directory"=w327:path)
            n138 = Build Path(base path=w327, name or relative path="MIDI\\midi_messages") -> (appended path=w336:path)
            n139 = Concatenate Strings(w326, ".txt" ("string")) -> (w333:string)
            n140 = Build Path(base path=w336, name or relative path=w333) -> (appended path=w332:path)
            n141 = Concatenate Strings("Saving Custom Message \"" ("string"), w326, "\". Data: " ("string")) -> (w323:string)
            n142 = Concatenate Strings(w323, w322) -> (w320:string)
            n143 = Open/Create/Replace File(file path (use dialog)=w332, error in=w328, operation (0:open)=T20."replace or create with confirmation", access (0:read/write)=enum16{"read/write", "read-only", "write-only"}."write-only") -> (refnum out=w340:refnum<file>, cancelled=w341:bool, error out=w339:errorcluster)  [unwired: 2 in]
            n144 = case "Aborted" shown="False" w341 {
              tunnel: w340 -> [w349 w351]
              tunnel: w339 -> [w348 w350]
              tunnel: [w347 w351] -> w337
              tunnel: [w346 w350] -> w338
              tunnel: w322 -> [w345 _]
              frame False {
                n145 = Write to Text File(file (use dialog)=w349, text=w345, error in=w348) -> (refnum out=w347:refnum<file>, error out=w346:errorcluster)  [unwired: 1 in, 1 out]
              }
              frame True {
                # "Aborted"
              }
            }
            n146 = Close File(refnum=w337, error in=w338) -> (error out=w321:errorcluster)  [unwired: 1 out]
            n147 = call "Console Entry.vi"("Error In"=w321, "Data In"=w330, "Console Entry"=w320) -> ("Data out"=w318:T6)  [unwired: 8 in]
            n148 = Unbundle By Name(w318) -> ("Function_Queue.Queue_MIDI_Handler"=w331:refnum<queue>)
            n149 = Enqueue Element(queue=w331, element=T18 {"Application State"=enum."MH Load Messages", "Payload"=variant} ("Application Message"), error in (no error)=w321) -> (error out=w319:errorcluster)  [unwired: 1 in, 2 out]
            n150 = call "Console Entry.vi"("Error In"=w319, "Data In"=w318, "Console Entry"="Message stored in MIDI\\midi_messages, MIDI Messages list reloaded.") -> ("Data out"=w317:T6)  [unwired: 8 in]
          }
          event "BtnG: Stop Button": Value Change {
            w360 = T18 {"Application State"=enum."Idle", "Payload"=variant}  # element
            # "Sending quit messages for all queue-recipients."
            n151 = event-data() -> ()  [unwired: 1 in, 1 out]
            n152 = Unbundle By Name(w355) -> ("Function_Queue.Queue_MIDI_Handler"=w365:refnum<queue>, "Function_Queue.Queue_Session"=w364:refnum<queue>, "Function_Queue.Queue_Producer"=w363:refnum<queue>, "Function_Queue.Queue_Consumer"=w362:refnum<queue>)
            n153 = Bundle By Name(cluster=w360, "Application State"=Application_State."Quit Message" ("Data_Type")) -> (w358:T18)
            n154 = Build Array(w365, w364, w363, w362) -> (w361:refnum<queue>[])
            n155 = for {
              tunnel: w361 -> [w369] mode=indexing
              tunnel: w358 -> [w368]
              shift-right: [w366] -> w352
              shift-left: w353 -> [w367]
              # "Sending Quit messages."
              n156 = Enqueue Element(queue=w369, element=w368, error in (no error)=w367) -> (error out=w366:errorcluster)  [unwired: 1 in, 2 out]
            }
            n157 = call "Console Entry.vi"("Error In"=w352, "Data In"=w355, "Console Entry"="Shutdown procedure initiated.") -> ("Data out"=w354:T6)  [unwired: 8 in]
          }
          event Application Instance Close {
            w378 = T18 {"Application State"=enum."Idle", "Payload"=variant}  # element
            # "Sending quit messages for all queue-recipients."
            n158 = event-data() -> ()  [unwired: 1 in, 1 out]
            n159 = Unbundle By Name(w373) -> ("Function_Queue.Queue_MIDI_Handler"=w383:refnum<queue>, "Function_Queue.Queue_Session"=w382:refnum<queue>, "Function_Queue.Queue_Producer"=w381:refnum<queue>, "Function_Queue.Queue_Consumer"=w380:refnum<queue>)
            n160 = Bundle By Name(cluster=w378, "Application State"=Application_State."Quit Message" ("Data_Type")) -> (w376:T18)
            n161 = Build Array(w383, w382, w381, w380) -> (w379:refnum<queue>[])
            n162 = for {
              tunnel: w379 -> [w387] mode=indexing
              tunnel: w376 -> [w386]
              shift-right: [w384] -> w370
              shift-left: w371 -> [w385]
              # "Sending Quit messages."
              n163 = Enqueue Element(queue=w387, element=w386, error in (no error)=w385) -> (error out=w384:errorcluster)  [unwired: 1 in, 2 out]
            }
            n164 = call "Console Entry.vi"("Error In"=w370, "Data In"=w373, "Console Entry"="Shutdown procedure initiated. Instance Close") -> ("Data out"=w372:T6)  [unwired: 8 in]
          }
          event "BtnG: Minimize": Value Change {
            n165 = event-data() -> ()  [unwired: 1 in, 6 out]
            n166 = control-ref of="This VI"() -> (w390:refnum<vi>)
            n167 = property class="VI"(reference=w390, error in=w391, "FP.State"=T16."Minimized" ("Front Panel Window:State")) -> (error out=w388:errorcluster)  [unwired: 1 out]
          }
          event Panel Close {
            w401 = T18 {"Application State"=enum."Idle", "Payload"=variant}  # element
            # "Sending quit messages for all queue-recipients."
            n168 = event-data() -> ()  [unwired: 1 in, 4 out]
            n169 = Unbundle By Name(w396) -> ("Function_Queue.Queue_MIDI_Handler"=w406:refnum<queue>, "Function_Queue.Queue_Session"=w405:refnum<queue>, "Function_Queue.Queue_Producer"=w404:refnum<queue>, "Function_Queue.Queue_Consumer"=w403:refnum<queue>)
            n170 = Bundle By Name(cluster=w401, "Application State"=Application_State."Quit Message" ("Data_Type")) -> (w399:T18)
            n171 = Build Array(w406, w405, w404, w403) -> (w402:refnum<queue>[])
            n172 = for {
              tunnel: w402 -> [w410] mode=indexing
              tunnel: w399 -> [w409]
              shift-right: [w407] -> w393
              shift-left: w394 -> [w408]
              # "Sending Quit messages."
              n173 = Enqueue Element(queue=w410, element=w409, error in (no error)=w408) -> (error out=w407:errorcluster)  [unwired: 1 in, 2 out]
            }
            n174 = call "Console Entry.vi"("Error In"=w393, "Data In"=w396, "Console Entry"="Shutdown procedure initiated. Panel Close") -> ("Data out"=w395:T6)  [unwired: 8 in]
          }
          event "BtnM: Update Settings": Value Change {
            w415 = T23 {"Tx Protocol"=enum."Not Active", "Rx Protocol"=enum."Serial", "Serial"={"Tx Port"="", "Rx Port"="", "Baud rate"=8, "Parity"=enum."None", "Data bits"=0, "Stop bits"=0, "Flow control"=enum."None", "Tx Resource"="", "Rx Resource"=""}, "MIDI Device"={"Input uDevice ID"=0, "Output uDevice ID"=0, "hmidiout Handle"=0, "hmidiin Handle"=0}, "Bluetooth"={"Dummy"=""}, "USB"={"Dummy"=""}}  # Com. Settings
            w425 = T18 {"Application State"=enum."Settings", "Payload"=variant}  # App Message
            # "It might be beneficial to place these clusters in the application data."
            # "Future Work:\n- Support for other connections"
            # "Updates Producer settings: Communication Protocol and Protocol Settings."
            n175 = event-data() -> ()  [unwired: 1 in, 1 out]
            n176 = Unbundle By Name(w420) -> ("Function_Queue.Queue_Producer"=w426:refnum<queue>)
            n177 = property on="BtnM: Initiate Producer" class="Bool"("DisabledEnum"=T17."Enabled" ("Disabled")) -> ()  [unwired: 2 in, 2 out]
            n178 = case "Tx Settings" shown="\"Serial\", Default" "Tx Protocol" {
              selector: "Tx Protocol" -> [w444 _ _ _ _]
              tunnel: w415 -> [w443 w448 w449 w450 w451]
              tunnel: [w438 w448 w449 w450 w451] -> w413
              tunnel: "Serial Communication" -> [w437 _ _ _ _]
              frame "Serial", Default {
                n179 = Unbundle By Name(w437) -> ("Baud rate"=w446:i32, "Tx Port"=w445:refnum<visa-resource-name>)
                n180 = Bundle By Name(cluster=w443, "Serial.Baud rate"=w446, "Serial.Tx Port"=w445, "Tx Protocol"=w444, "Serial.Parity"=enum16{"None", "Odd", "Even", "Mark", "Space"}."None", "Serial.Data bits"=8, "Serial.Stop bits"=10, "Serial.Flow control"=T21."None", "Serial.Tx Resource"=refnum<visa-resource-name> refnum) -> (w438:T23)
              }
              frame "Bluetooth" {
              }
              frame "USB-MIDI" {
              }
              frame "MIDI (Audio Device)" {
              }
              frame "Not Active" {
              }
            }
            n181 = case "Rx Settings" shown="\"Serial\", Default" "Rx Protocol" {
              selector: "Rx Protocol" -> [w432 _ _ _ _]
              tunnel: w413 -> [w431 w433 w434 w435 w436]
              tunnel: [w430 w433 w434 w435 w436] -> w412
              tunnel: "Serial Communication" -> [w429 _ _ _ _]
              frame "Serial", Default {
                n182 = Unbundle By Name(w429) -> ("Rx Port"=w428:refnum<visa-resource-name>)
                n183 = Bundle By Name(cluster=w431, "Serial.Rx Port"=w428, "Rx Protocol"=w432, "Serial.Rx Resource"=refnum<visa-resource-name> refnum) -> (w430:T23)
              }
              frame "Bluetooth" {
              }
              frame "USB-MIDI" {
              }
              frame "MIDI (Audio Device)" {
              }
              frame "Not Active" {
              }
            }
            n184 = Bundle By Name(cluster=w425, "Payload"=w412) -> (w424:T18)
            n185 = Enqueue Element(queue=w426, element=w424, error in (no error)=w418) -> (error out=w417:errorcluster)  [unwired: 1 in, 2 out]
            n186 = call "Console Entry.vi"("Error In"=w417, "Data In"=w420, "Console Entry"="Updating communication settings.") -> ("Data out"=w419:T6)  [unwired: 8 in]
          }
          event "BtnMS: Compose Message": Value Change {
            w460 = T17."Disabled and Grayed Out" ("Disabled")
            w462 = T17."Enabled" ("Disabled")
            w467 = T9 []  # MIDI Message Array
            # "Composes array of messages and transfers them to Producer. Producer Session is Initiated, Session GUI-tab is opened with \"Prod-Session.vi\". Session is started by user."
            n187 = event-data() -> ()  [unwired: 1 in, 1 out]
            n188 = property on="List: Send" class="LstBox (strict)"() -> ("Item Names"=w481:string[])  [unwired: 2 in, 2 out]
            n189 = Unbundle By Name "Buffered Messages"(w458) -> ("MIDI-Messages"=w479:T9)
            n190 = property on="List: MIDI Messages" class="LstBox (strict)"() -> ("Item Names"=w480:string[])  [unwired: 2 in, 2 out]
            n191 = for "Search for Message & Content" {
              tunnel: w481 -> [w492] mode=indexing
              tunnel: w480 -> [w491]
              tunnel: w479 -> [w490]
              shift-right: [w487] -> w470
              shift-left: w467 -> [w488]
              shift-right: [w482] -> w468
              shift-left: w469 -> [w483]
              # "Search Buffered Message list for Send-items"
              n192 = Search 1D Array(1D array=w491, element=w492) -> (index of element=w486:i32)  [unwired: 1 in]
              n193 = Equal?(x=w486, y=-1) -> (x = y?=w484:bool)
              n194 = Index Array(array=w490, index=w486) -> (element=w489:T10)
              n195 = Insert Into Array(array=w488, new element=w489) -> (w487:T9)  [unwired: 1 in]
              n196 = case "Message not found" shown="True" w484 {
                tunnel: w483 -> [w493 _]
                tunnel: [w493 errorcluster {"status"=TRUE, "code"=0, "source"="Custom Error: Message not found! \"No Data\"-type?"} ("error IO")] -> w482
                frame False {
                }
                frame True {
                }
              }
            }
            n197 = property on="BtnS: Pause Session" class="Bool"("DisabledEnum"=w460, "BoolText.Text"="Not Active" ("Boolean Text.Text")) -> ()  [unwired: 2 in, 2 out]
            n198 = property on="BtnSI: Inspect Session" class="Bool"("DisabledEnum"=w460, "BoolText.Text"="No Data" ("Boolean Text.Text")) -> ()  [unwired: 2 in, 2 out]
            n199 = property on="BtnS: Start/Resume Session" class="Bool"("Blinking"=FALSE, "DisabledEnum"=w462, "BoolText.Text"="Start Session" ("Boolean Text.Text")) -> ()  [unwired: 2 in, 2 out]
            n200 = property on="BtnS: Stop Session" class="Bool"("DisabledEnum"=w462, "BoolText.Text"="Abort" ("Boolean Text.Text")) -> ()  [unwired: 2 in, 2 out]
            n201 = property on="GUI Tab" class="TabCtl (strict)"("Value"=T1."Session GUI" ("GUI Tab")) -> ()  [unwired: 2 in, 2 out]
            n202 = Bundle By Name(cluster=T18 {"Application State"=enum."Com Session", "Payload"=variant} ("Application Message"), "Payload"=w470) -> (w471:T18)
            n203 = Unbundle By Name(w458) -> ("Function_Queue.Queue_Producer"=w472:refnum<queue>)
            n204 = Enqueue Element(queue=w472, element=w471, error in (no error)=w468) -> (error out=w455:errorcluster)  [unwired: 1 in, 2 out]
            n205 = vi-ref "Prod - Session.vi"() -> (w453:refnum<vi>)
            n206 = Bundle By Name(cluster=w458, "Com Session State"=Session_State."Wait to begin") -> (w457:T6)
            n207 = invoke on="Prod - Session.vi" class="SubPnl" method="Insert VI"(error in=w455, "VI Ref"=w453) -> (error out=w454:errorcluster)  [unwired: 2 in, 3 out]
            n208 = Array Size(array=w470) -> (size(s)=w478:i32)
            n209 = Number To Decimal String(number=w478) -> (decimal integer string=w475:string)  [unwired: 1 in]
            n210 = Concatenate Strings("Processing " ("string"), w475, " messages/commandos to send. " ("string")) -> (w474:string)
            n211 = call "Console Entry.vi"("Error In"=w454, "Data In"=w457, "Console Entry"=w474) -> ("Data out"=w473:T6)  [unwired: 8 in]
          }
          event "BtnM: All": Value Change {
            n212 = event-data() -> ()  [unwired: 1 in, 6 out]
            n213 = call <vilib>:"Application Directory.vi"() -> ("Application Directory"=w516:path)
            n214 = Build Path(base path=w516, name or relative path="MIDI\\standardized_tests") -> (appended path=w514:path)
            n215 = Build Path(base path=w514, name or relative path="all_messages.txt") -> (appended path=w512:path)
            n216 = Open/Create/Replace File(file path (use dialog)=w512, error in=w519, operation (0:open)=T20."open", access (0:read/write)=enum16{"read/write", "read-only", "write-only"}."read-only") -> (refnum out=w517:refnum<file>, error out=w518:errorcluster)  [unwired: 2 in, 1 out]
            n217 = Read from Text File(file (use dialog)=w517, error in=w518) -> (text=w506:string, error out=w500:errorcluster)  [unwired: 2 in, 2 out]
            n218 = String Length(string=w506) -> (length=w509:i32)
            n219 = Quotient & Remainder(x=w509, y=1499) -> (floor(x/y)=w507:i32)  [unwired: 1 out]
            n220 = Increment(x=w507) -> (x+1=w505:i32)
            n221 = for {
              N: w505 -> [_]
              shift-right: [w539] -> _
              shift-left: w506 -> [w541]
              shift-right: [w530] -> w501
              shift-left: T9 [] ("MIDI Message Array") -> [w531]
              tunnel: [w520] -> w495 mode=concatenating
              i -> [w535]
              w526 = 10  # Delay
              w521 = "Delay 10ms" ("Message Name")
              w528 = T10 {"Message Name"="", "Meta value"=0, "Datastring"="", "Datatype"=enum."Pause"} ("MIDI Message Cluster")
              n222 = Increment(x=w535) -> (x+1=w534:i32)
              n223 = String Subset(string=w541, offset (0)=0, length (rest)=2998 ("length (rest)")) -> (substring=w533:string)
              n224 = String Subset(string=w541, offset (0)=2998) -> (substring=w539:string)  [unwired: 1 in]
              n225 = Number To Decimal String(number=w534) -> (decimal integer string=w538:string)  [unwired: 1 in]
              n226 = Concatenate Strings("All (" ("string"), w538, ")" ("string")) -> (w522:string)
              n227 = Bundle By Name(cluster=w528, "Message Name"=w522, "Meta value"=0, "Datastring"=w533, "Datatype"=Meta_Commands."MIDI") -> (w529:T10)
              n228 = Bundle By Name(cluster=w528, "Message Name"=w521, "Meta value"=w526, "Datastring"="", "Datatype"=Meta_Commands."Delay") -> (w527:T10)
              n229 = Build Array(w522, w521) -> (w520:string[])
              n230 = Insert Into Array(array=w531, new element #1=w529, new element #2=w527) -> (w530:T9)  [unwired: 1 in]
            }
            n231 = property on="List: MIDI Messages" class="LstBox (strict)"() -> (error out=w496:errorcluster, "Item Names"=w498:string[])  [unwired: 2 in, 1 out]
            n232 = Insert Into Array(array=w498, new element=w495) -> (w497:string[])  [unwired: 1 in]
            n233 = property on="List: Send" class="LstBox (strict)"("Item Names"=w495) -> ()  [unwired: 2 in, 2 out]
            n234 = Bundle By Name(cluster=w502, "MIDI-Messages"=w501) -> (w503:T6)
            n235 = property on="List: MIDI Messages" class="LstBox (strict)"(error in=w496, "Item Names"=w497) -> ()  [unwired: 1 in, 2 out]
          }
          event "BtnS: Pause Session": Value Change {
            w549 = Session_State."Pause" ("Enum")
            w555 = T17."Disabled and Grayed Out" ("Disabled")
            w557 = T17."Enabled" ("Disabled")
            # "Pauses the Producer Session, Rx is still active."
            n236 = event-data() -> ()  [unwired: 1 in, 1 out]
            n237 = Unbundle By Name(w550) -> ("Function_Queue.Queue_Session"=w553:refnum<queue>)
            n238 = Bundle By Name(cluster=T18 {"Application State"=enum."Idle", "Payload"=variant} ("element"), "Payload"=w549) -> (w551:T18)
            n239 = Enqueue Element(queue=w553, element=w551, error in (no error)=w548) -> (error out=w544:errorcluster)  [unwired: 1 in, 2 out]
            n240 = Bundle By Name(cluster=w550, "Com Session State"=w549) -> (w546:T6)
            n241 = property on="BtnS: Start/Resume Session" class="Bool"("Blinking"=FALSE, "DisabledEnum"=w557, "BoolText.Text"="Resume Session" ("Boolean Text.Text")) -> ()  [unwired: 2 in, 2 out]
            n242 = property on="BtnS: Stop Session" class="Bool"("DisabledEnum"=w557, "BoolText.Text"="Stop Session" ("Boolean Text.Text")) -> ()  [unwired: 2 in, 2 out]
            n243 = property on="BtnS: Pause Session" class="Bool"("DisabledEnum"=w555, "BoolText.Text"="Paused" ("Boolean Text.Text")) -> ()  [unwired: 2 in, 2 out]
            n244 = property on="BtnSI: Inspect Session" class="Bool"("DisabledEnum"=w555, "BoolText.Text"="Stop first" ("Boolean Text.Text")) -> ()  [unwired: 2 in, 2 out]
            n245 = call "Console Entry.vi"("Error In"=w544, "Data In"=w546, "Console Entry"="Producer pausing.") -> ("Data out"=w545:T6)  [unwired: 8 in]
          }
          event "BtnS: Start/Resume Session": Value Change {
            w573 = T17."Disabled and Grayed Out" ("Disabled")
            # "Producer Session Start/Resume/Restart based on Session State."
            n246 = event-data() -> ()  [unwired: 1 in, 1 out]
            n247 = Unbundle By Name(w563) -> ("Com Session State"=w567:T11)
            n248 = property on="BtnS: Pause Session" class="Bool"("DisabledEnum"=T17."Enabled" ("Disabled"), "BoolText.Text"="Pause" ("Boolean Text.Text")) -> ()  [unwired: 2 in, 2 out]
            n249 = property on="BtnS: Start/Resume Session" class="Bool"("Blinking"=TRUE, "DisabledEnum"=w573, "BoolText.Text"="Session Active" ("Boolean Text.Text")) -> ()  [unwired: 2 in, 2 out]
            n250 = property on="BtnS: Stop Session" class="Bool"("DisabledEnum"=w573, "BoolText.Text"="Pause first" ("Boolean Text.Text")) -> ()  [unwired: 2 in, 2 out]
            n251 = property on="BtnSI: Inspect Session" class="Bool"("DisabledEnum"=w573, "BoolText.Text"="Stop first" ("Boolean Text.Text")) -> ()  [unwired: 2 in, 2 out]
            n252 = case shown="\"Stop\"" w567 {
              tunnel: [Session_State."Active Session" ("Enum") Session_State."Active Session" ("Enum") Session_State."Active Session" ("Enum") Session_State."Active Session" ("Enum")] -> w566
              tunnel: [Session_State."Active Session" ("Enum") Session_State."Active Session" ("Enum") Session_State."Active Session" ("Enum") Session_State."Restart" ("Enum")] -> w565
              tunnel: ["Session started" ("Console Entry") "Session resumed" ("Console Entry") "User resumed session, after \"wait for Rx\". " ("Console Entry") "Session restarted." ("Console Entry")] -> w564
              frame "Wait to begin", Default {
                # "Initial function"
              }
              frame "Pause" {
              }
              frame "Wait for Response" {
              }
              frame "Stop" {
              }
            }
            n253 = Unbundle By Name(w563) -> ("Function_Queue.Queue_Session"=w572:refnum<queue>)
            n254 = Bundle By Name(cluster=T18 {"Application State"=enum."Idle", "Payload"=variant} ("element"), "Payload"=w565) -> (w570:T18)
            n255 = call "Console Entry.vi"("Error In"=w561, "Data In"=w563, "Console Entry"=w564) -> ("Data out"=w562:T6)  [unwired: 8 in]
            n256 = Enqueue Element(queue=w572, element=w570, error in (no error)=w561) -> (error out=w568:errorcluster)  [unwired: 1 in, 2 out]
            n257 = Bundle By Name(cluster=w562, "Com Session State"=w566) -> (w569:T6)
          }
          event "BtnS: Stop Session": Value Change {
            # "Change state in session VI."
            # "Abort, Stop or Exit Producer Session based upon which state the session is in."
            n258 = event-data() -> ()  [unwired: 1 in, 1 out]
            n259 = Unbundle By Name(w598) -> ("Com Session State"=w600:T11)
            n260 = case shown="\"Stop\"" w600 {
              tunnel: [Session_State."Exit" ("Com Session State") Session_State."Stop" ("Com Session State") Session_State."Stop" ("Com Session State") Session_State."Exit" ("Com Session State")] -> w597
              tunnel: w596 -> [w607 w610 w620 w625]
              tunnel: [w606 w610 w620 w624] -> w594
              tunnel: ["Session aborted." "Session stopped." "User stopped Session after \"Wait for Rx\"." "Exit Session."] -> w593
              frame "Wait to begin", Default {
                # "Session hasn't started yet, button says abort."
                n261 = property on="GUI Tab" class="TabCtl (strict)"("Value"=T1."Main GUI" ("GUI Tab")) -> ()  [unwired: 2 in, 2 out]
                n262 = invoke on="Prod - Session.vi" class="SubPnl" method="Remove VI"(error in=w607) -> (error out=w606:errorcluster)  [unwired: 2 in, 2 out]
              }
              frame "Pause" {
                w617 = T17."Enabled" ("Disabled")
                # "Session Paused"
                n263 = property on="BtnS: Start/Resume Session" class="Bool"("Blinking"=FALSE, "DisabledEnum"=w617, "BoolText.Text"="Restart Session" ("Boolean Text.Text")) -> ()  [unwired: 2 in, 2 out]
                n264 = property on="BtnS: Stop Session" class="Bool"("DisabledEnum"=w617, "BoolText.Text"="Exit" ("Boolean Text.Text")) -> ()  [unwired: 2 in, 2 out]
                n265 = property on="BtnSI: Inspect Session" class="Bool"("DisabledEnum"=w617, "BoolText.Text"="Inspect Data" ("Boolean Text.Text")) -> ()  [unwired: 2 in, 2 out]
                n266 = property on="BtnS: Pause Session" class="Bool"("DisabledEnum"=T17."Disabled and Grayed Out" ("Disabled"), "BoolText.Text"="Not Active" ("Boolean Text.Text")) -> ()  [unwired: 2 in, 2 out]
              }
              frame "Wait for Response" {
                # "The Session is waiting for 100% throughput"
              }
              frame "Stop" {
                # "The Program is stopped, and button says exit."
                n267 = property on="GUI Tab" class="TabCtl (strict)"("Value"=T1."Main GUI" ("GUI Tab")) -> ()  [unwired: 2 in, 2 out]
                n268 = invoke on="Prod - Session.vi" class="SubPnl" method="Remove VI"(error in=w625) -> (error out=w624:errorcluster)  [unwired: 2 in, 2 out]
              }
            }
            n269 = Bundle By Name(cluster=w598, "Com Session State"=w597) -> (w595:T6)
            n270 = call "Console Entry.vi"("Error In"=w594, "Data In"=w595, "Console Entry"=w593) -> ("Data out"=w592:T6)  [unwired: 8 in]
            n271 = Unbundle By Name(w592) -> ("Function_Queue.Queue_Session"=w603:refnum<queue>)
            n272 = Bundle By Name(cluster=T18 {"Application State"=enum."Idle", "Payload"=variant} ("element"), "Payload"=w597) -> (w602:T18)
            n273 = Enqueue Element(queue=w603, element=w602, error in (no error)=w594) -> (error out=w599:errorcluster)  [unwired: 1 in, 2 out]
          }
          event "BtnSI: Inspect Session": Value Change {
            w636 = Session_State."Inspect" ("Enum")
            # "Changes the GUI-tab to Inspect. Session.vi Closed."
            n274 = event-data() -> ()  [unwired: 1 in, 1 out]
            n275 = Unbundle By Name(w634) -> ("Function_Queue.Queue_Session"=w638:refnum<queue>)
            n276 = property on="GUI Tab" class="TabCtl (strict)"("Value"=T1."Inspect GUI" ("GUI Tab")) -> ()  [unwired: 2 in, 2 out]
            n277 = Bundle By Name(cluster=T18 {"Application State"=enum."Idle", "Payload"=variant} ("element"), "Payload"=w636) -> (w637:T18)
            n278 = Enqueue Element(queue=w638, element=w637, error in (no error)=w632) -> (error out=w633:errorcluster)  [unwired: 1 in, 2 out]
            n279 = invoke on="Prod - Session.vi" class="SubPnl" method="Remove VI"(error in=w633) -> (error out=w631:errorcluster)  [unwired: 2 in, 2 out]
            n280 = Bundle By Name(cluster=w634, "Com Session State"=w636) -> (w628:T6)
            n281 = call "Console Entry.vi"("Data In"=w628, "Console Entry"="Session finished, Inspection initiated.") -> ("Data out"=w630:T6)  [unwired: 9 in]
          }
          event "BtnI: Inspect Parsing": Value Change {
            n282 = event-data() -> ()  [unwired: 1 in, 1 out]
            n283 = property on="GUI Tab" class="TabCtl (strict)"(error in=w640, "Value"=T1."Parsing" ("GUI Tab")) -> (error out=w639:errorcluster)  [unwired: 1 in, 1 out]
          }
          event "Custom Message.Message Name": Drop {
            # "Populates the \"Custom Message\" by dropping an item from the \"MIDI Messages\"-list to the \"Message Name\" in \"Custom Message\". The value of populated fields are the same as the item."
            n284 = event-data() -> ()  [unwired: 1 in, 1 out]
            n285 = Unbundle By Name(w646) -> ("MIDI-Messages"=w653:T9)
            n286 = property on="List: MIDI Messages" class="LstBox (strict)"(error in=w647) -> (error out=w650:errorcluster, "Item Names"=w655:string[], "FocusRow"=w648:i32)  [unwired: 1 in, 1 out]
            n287 = Index Array(array=w653, index=w648) -> (element=w652:T10)
            n288 = Index Array(array=w655, index=w648) -> (element=w654:string)
            n289 = property on="Message Name" class="Str"(error in=w650, "Value"=w654) -> (error out=w649:errorcluster)  [unwired: 1 in, 1 out]
            n290 = Unbundle By Name(w652) -> ("Datastring"=w651:string)
            n291 = property on="Message Data" class="Str"(error in=w649, "Value"=w651) -> (error out=w644:errorcluster)  [unwired: 1 in, 1 out]
            n292 = event-data() -> ()  [unwired: 2 in, 1 out]
            n293 = call "Console Entry.vi"("Error In"=w644, "Data In"=w646, "Console Entry"="Inspecting MIDI-message in Custom Message.") -> ("Data out"=w645:T6)  [unwired: 8 in]
          }
          event "Data error?": Mouse Down {
            # "Transports the user to the first row containing a data error."
            n294 = event-data() -> ()  [unwired: 1 in, 1 out]
            n295 = property on="Diff" class="Arr (strict)"(error in=w661) -> (error out=w660:errorcluster, "Index Values"=w668:u32[])  [unwired: 1 in, 1 out]
            n296 = Index Array(array=w668, index=0) -> (element=w666:u32)
            n297 = Unbundle By Name(w658) -> ("Result Data.Diff"=w669:bool[])
            n298 = Search 1D Array(1D array=w669, element=TRUE, start index (0)=w666) -> (index of element=w663:i32)
            n299 = Decrement(x=w663) -> (x-1=w662:i32)
            n300 = Initialize Array(w662, 1 ("dimension size")) -> (w664:i32[])
            n301 = property on="Scrollbar" class="Scroll (strict)"(error in=w660, "Value"=w662) -> (error out=w656:errorcluster)  [unwired: 1 in, 1 out]
            n302 = property on="Send Log" class="Arr (strict)"("Index Values"=w664) -> ()  [unwired: 2 in, 2 out]
            n303 = property on="Tx Log" class="Arr (strict)"("Index Values"=w664) -> ()  [unwired: 2 in, 2 out]
            n304 = property on="Rx Log" class="Arr (strict)"("Index Values"=w664) -> ()  [unwired: 2 in, 2 out]
            n305 = property on="Diff" class="Arr (strict)"("Index Values"=w664) -> ()  [unwired: 2 in, 2 out]
            n306 = property on="Get #" class="Arr (strict)"("Index Values"=w664) -> ()  [unwired: 2 in, 2 out]
            n307 = call "Console Entry.vi"("Error In"=w656, "Data In"=w658, "Console Entry"="Scroll transported to first error cell.") -> ("Data out"=w659:T6)  [unwired: 8 in]
          }
          event "Get #": Value Change {
            # "Gets the row number of clicked cell. To easier reference it in data-loss correction."
            n308 = event-data() -> ()  [unwired: 1 in, 1 out]
            n309 = Array Size(array="Get #") -> (size(s)=w685:i32)
            n310 = Search 1D Array(1D array="Get #", element=TRUE, start index (0)=0) -> (index of element=w676:i32)
            "Get #" <- w676
            n311 = Initialize Array(FALSE, w685) -> (w684:bool[])
            n312 = property on="Get #" class="Arr (strict)"(error in=w680, "Value"=w684) -> (error out=w672:errorcluster)  [unwired: 1 in, 1 out]
            n313 = Number To Decimal String(number=w676) -> (decimal integer string=w677:string)  [unwired: 1 in]
            n314 = Concatenate Strings("Get cell: ", w677, ".") -> (w675:string)
            n315 = call "Console Entry.vi"("Error In"=w672, "Data In"=w674, "Console Entry"=w675) -> ("Data out"=w673:T6)  [unwired: 8 in]
          }
          event "List: MIDI Messages": Double Click {
            # "Adds double clicked item to the  Send-list."
            n316 = event-data() -> ("Row"=w698:i32)  [unwired: 1 in]
            n317 = property on="List: MIDI Messages" class="LstBox (strict)"(error in=w696) -> (error out=w695:errorcluster, "Item Names"=w699:string[])  [unwired: 1 in, 1 out]
            n318 = property on="List: Send" class="LstBox (strict)"(error in=w695) -> (error out=w694:errorcluster, "Item Names"=w700:string[])  [unwired: 1 in, 1 out]
            n319 = Index Array(array=w699, index=w698) -> (element=w691:string)
            n320 = Insert Into Array(array=w700, new element=w691) -> (w697:string[])  [unwired: 1 in]
            n321 = property on="List: Send" class="LstBox (strict)"(error in=w694, "Item Names"=w697) -> (error out=w689:errorcluster)  [unwired: 1 in, 1 out]
            n322 = Concatenate Strings("Added \"" ("string"), w691, "\" to Send-list." ("string")) -> (w693:string)
            n323 = call "Console Entry.vi"("Error In"=w689, "Data In"=w690, "Console Entry"=w693) -> ("Data out"=w687:T6)  [unwired: 8 in]
          }
          event "List: Send": Double Click {
            # "Deletes the item double clicked from the Send-list"
            n324 = event-data() -> ("Row"=w712:i32)  [unwired: 1 in]
            n325 = property on="List: Send" class="LstBox (strict)"(error in=w707) -> (error out=w706:errorcluster, "Item Names"=w711:string[])  [unwired: 1 in, 1 out]
            n326 = Delete From Array(array=w711, index=w712) -> (deleted portion=w705:string, array with subset deleted=w710:string[])  [unwired: 1 in]
            n327 = property on="List: Send" class="LstBox (strict)"(error in=w706, "Item Names"=w710) -> (error out=w701:errorcluster)  [unwired: 1 in, 1 out]
            n328 = Concatenate Strings("Deleted \"" ("string"), w705, "\" from the Send-list." ("string")) -> (w704:string)
            n329 = call "Console Entry.vi"("Error In"=w701, "Data In"=w703, "Console Entry"=w704) -> ("Data out"=w702:T6)  [unwired: 8 in]
          }
          event "Scrollbar", "Scrollbar Parse": Value Change {
            n330 = event-data() -> ()  [unwired: 1 in, 1 out]
            n331 = Initialize Array("Scrollbar", 1 ("dimension size")) -> (w718:i32[])
            n332 = property on="Send Log" class="Arr (strict)"(error in=w717, "Index Values"=w718) -> (error out=w716:errorcluster)  [unwired: 1 in, 1 out]
            n333 = property on="Tx Log" class="Arr (strict)"("Index Values"=w718) -> ()  [unwired: 2 in, 2 out]
            n334 = property on="Rx Log" class="Arr (strict)"("Index Values"=w718) -> ()  [unwired: 2 in, 2 out]
            n335 = property on="Diff" class="Arr (strict)"("Index Values"=w718) -> ()  [unwired: 2 in, 2 out]
            n336 = property on="Get #" class="Arr (strict)"("Index Values"=w718) -> ()  [unwired: 2 in, 2 out]
            n337 = Initialize Array("Scrollbar Parse", 1 ("dimension size")) -> (w713:i32[])
            n338 = property on="Tx Running States" class="Arr (strict)"("Index Values"=w713) -> ()  [unwired: 2 in, 2 out]
            n339 = property on="Tx Error?" class="Arr (strict)"("Index Values"=w713) -> ()  [unwired: 2 in, 2 out]
            n340 = property on="Tx MIDI Message Type" class="Arr (strict)"("Index Values"=w713) -> ()  [unwired: 2 in, 2 out]
            n341 = property on="Tx Parsed Data" class="Arr (strict)"("Index Values"=w713) -> ()  [unwired: 2 in, 2 out]
            n342 = property on="Diff" class="Arr (strict)"("Index Values"=w713) -> ()  [unwired: 2 in, 2 out]
            n343 = property on="Rx Parsed Data" class="Arr (strict)"("Index Values"=w713) -> ()  [unwired: 2 in, 2 out]
            n344 = property on="Rx MIDI Message Type" class="Arr (strict)"("Index Values"=w713) -> ()  [unwired: 2 in, 2 out]
            n345 = property on="Rx Error?" class="Arr (strict)"("Index Values"=w713) -> ()  [unwired: 2 in, 2 out]
            n346 = property on="Rx Running States" class="Arr (strict)"("Index Values"=w713) -> ()  [unwired: 2 in, 2 out]
          }
          event User Event {
            # "RAM"
            # "Imports Data from Inspect.vi, which was tranfered from the Producer Session."
            n347 = event-data() -> ("Payload"=w760:variant)  [unwired: 1 in]
            n348 = Variant To Data(error in=w759, type=T12 {"Diff"=[], "Tx Byte"=[], "Rx Byte"=[], "Send Log"=[], "Parsed Data"={"Tx MIDI Tag"=[], "Tx MIDI Parsed Data"=[], "Tx Error"=[], "Tx Running States"=[], "Rx MIDI Tag"=[], "Rx MIDI Parsed Data"=[], "Rx Error"=[], "Rx Running States"=[], "Diff"=[]}}, Variant=w760) -> (data=w727:T12, error out=w740:errorcluster)
            n349 = Unbundle By Name(w727) -> ("Parsed Data.Rx Error"=w724:bool[], "Parsed Data.Tx Error"=w723:bool[])
            n350 = Unbundle By Name(w727) -> ("Tx Byte"=w751:string[], "Rx Byte"=w750:string[], "Diff"=w746:bool[])
            n351 = Boolean To (0,1)(Boolean=w746) -> (0, 1=w745:i16[])
            n352 = Array Size(array=w724) -> (size(s)=w726:i32)
            n353 = Array Size(array=w723) -> (size(s)=w725:i32)
            n354 = Array Size(array=w751) -> (size(s)=w749:i32)
            n355 = Array Size(array=w750) -> (size(s)=w748:i32)
            n356 = Or Array Elements(Boolean array=w746) -> (logical OR=→"Data error?":bool)
            n357 = Array Size(array=w746) -> (size(s)=w755:i32)
            n358 = Max & Min(x=w726, y=w725) -> (max(x,y)=w722:i32)  [unwired: 1 out]
            n359 = Subtract(x=w749, y=w748) -> (x-y=→"Bytes lost":i32)
            n360 = property on="Scrollbar" class="Scroll (strict)"(error in=w740, "Value"=0 ("Scrollbar"), "DocMax"=w755) -> (error out=w739:errorcluster)  [unwired: 1 in, 1 out]
            n361 = Add Array Elements(numeric array=w745) -> (sum=→"Diff bytes":i16)
            n362 = Initialize Array(FALSE, w755) -> (w752:bool[])
            n363 = property on="Get #" class="Arr (strict)"(error in=w739, "Value"=w752) -> (error out=w738:errorcluster)  [unwired: 1 in, 1 out]
            n364 = Initialize Array(0 ("element"), 1 ("dimension size")) -> (w743:i32[])
            n365 = property on="Send Log" class="Arr (strict)"("Index Values"=w743) -> ()  [unwired: 2 in, 2 out]
            n366 = property on="Tx Log" class="Arr (strict)"("Index Values"=w743) -> ()  [unwired: 2 in, 2 out]
            n367 = property on="Rx Log" class="Arr (strict)"("Index Values"=w743) -> ()  [unwired: 2 in, 2 out]
            n368 = property on="Diff" class="Arr (strict)"("Index Values"=w743) -> ()  [unwired: 2 in, 2 out]
            n369 = property on="Get #" class="Arr (strict)"(error in=w738, "Index Values"=w743) -> (error out=w728:errorcluster)  [unwired: 1 in, 1 out]
            n370 = property on="Scrollbar Parse" class="Scroll (strict)"(error in=w728, "Value"=0 ("Scrollbar Parse"), "DocMax"=w722) -> (error out=w729:errorcluster)  [unwired: 1 in, 1 out]
            n371 = Bundle By Name(cluster=w753, "Result Data"=w727, "Get #"=w752) -> (w737:T6)
            n372 = Initialize Array(0 ("element"), 1 ("dimension size")) -> (w732:i32[])
            n373 = property on="Tx Running States" class="Arr (strict)"("Index Values"=w732) -> ()  [unwired: 2 in, 2 out]
            n374 = property on="Tx Error?" class="Arr (strict)"("Index Values"=w732) -> ()  [unwired: 2 in, 2 out]
            n375 = property on="Tx MIDI Message Type" class="Arr (strict)"("Index Values"=w732) -> ()  [unwired: 2 in, 2 out]
            n376 = property on="Tx Parsed Data" class="Arr (strict)"("Index Values"=w732) -> ()  [unwired: 2 in, 2 out]
            n377 = property on="Diff" class="Arr (strict)"("Index Values"=w732) -> ()  [unwired: 2 in, 2 out]
            n378 = property on="Rx Parsed Data" class="Arr (strict)"("Index Values"=w732) -> ()  [unwired: 2 in, 2 out]
            n379 = property on="Rx MIDI Message Type" class="Arr (strict)"("Index Values"=w732) -> ()  [unwired: 2 in, 2 out]
            n380 = property on="Rx Error?" class="Arr (strict)"("Index Values"=w732) -> ()  [unwired: 2 in, 2 out]
            n381 = property on="Rx Running States" class="Arr (strict)"(error in=w729, "Index Values"=w732) -> (error out=w731:errorcluster)  [unwired: 1 in, 1 out]
            n382 = call "Console Entry.vi"("Error In"=w731, "Data In"=w737, "Console Entry"="Session imported from Producer Session, after being treated by Inspector.") -> ("Data out"=w736:T6)  [unwired: 8 in]
          }
          event User Event {
            # "Error message from another VI."
            n383 = event-data() -> ("Payload"=w770:variant)  [unwired: 1 in, 4 out]
            n384 = Variant To Data(error in=w769, type="", Variant=w770) -> (data=w765:string, error out=w761:errorcluster)
            n385 = feedback #1("") -> (w772:string)
            n386 = Concatenate Strings(w772, w765) -> (w767:string)
            "Error Loop" <- w767
            n387 = feedback-in #1(w767) -> ()
            n388 = Concatenate Strings("An error has occured in another VI: " ("string"), w765) -> (w764:string)
            n389 = call "Console Entry.vi"("Error In"=w761, "Data In"=w763, "Console Entry"=w764) -> ("Data out"=w762:T6)  [unwired: 8 in]
          }
          event User Event {
            # "Response to \"Load Messages\"-event, returns available MIDI-messages from folder."
            n390 = event-data() -> ("Payload"=w783:variant)  [unwired: 1 in]
            n391 = Unbundle By Name(w779) -> ("MIDI-Messages"=w781:T9)
            n392 = Variant To Data(error in=w782, type=w781, Variant=w783) -> (data=w778:T9, error out=w774:errorcluster)
            n393 = Bundle By Name(cluster=w779, "MIDI-Messages"=w778) -> (w776:T6)
            n394 = for {
              tunnel: w778 -> [w785] mode=indexing
              tunnel: [w784] -> w780 mode=indexing
              n395 = Unbundle By Name(w785) -> ("Message Name"=w784:string)
            }
            n396 = property on="List: MIDI Messages" class="LstBox (strict)"("Item Names"=w780) -> ()  [unwired: 2 in, 2 out]
            n397 = call "Console Entry.vi"("Error In"=w774, "Data In"=w776, "Console Entry"="MIDI-messages loaded.") -> ("Data out"=w775:T6)  [unwired: 8 in]
          }
          event User Event {
            n398 = event-data() -> ("Payload"=w797:variant)  [unwired: 1 in]
            n399 = Variant To Data(error in=w795, type=T22 {"Datatype"=[], "Bytesize"=[], "Strings"=[], "ByteSum"=0} ("Tx Info"), Variant=w797) -> (data=w794:T22, error out=w788:errorcluster)
            n400 = Unbundle By Name(w794) -> ("Datatype"=→"Datatype":T5[], "Bytesize"=→"Bytesize":i32[], "Strings"=→"Strings":string[], "ByteSum"=→"Total amount of bytes to send":i32)
            n401 = call "Console Entry.vi"("Error In"=w788, "Data In"=w787, "Console Entry"="MIDI-messages compiled for TX, and pre-session Data returned from Producer Session.") -> ("Data out"=w789:T6)  [unwired: 8 in]
          }
          event User Event {
            n402 = event-data() -> ("Payload"=w806:variant)  [unwired: 1 in]
            n403 = Variant To Data(error in=w804, type=Session_State."Wait to begin" ("Enum"), Variant=w806) -> (data=w802:T11, error out=w799:errorcluster)
            n404 = Bundle By Name(cluster=w803, "Com Session State"=w802) -> (w800:T6)
            n405 = case shown="\"Pause\"" w802 {
              tunnel: ["Session paused by Tx-Producer, waiting for user input." "Session paused by Tx-Producer, waiting for Rx-data." "Session stopped by Tx-Producer. Should it be able to do that?" "An unexpeted Session state has occured: Restart." "An unexpeted Session state has occured: Inspect." "An unexpeted Session state has occured: Exit." "An unexpeted Session state has occured: Active Session." "An unexpeted Session state has occured: Wait to begin."] -> w798
              frame "Pause" {
                w814 = T17."Disabled and Grayed Out" ("Disabled")
                w812 = T17."Enabled" ("Disabled")
                # "Session paused, Rx still running."
                n406 = property on="BtnS: Start/Resume Session" class="Bool"("Blinking"=FALSE, "DisabledEnum"=w812, "BoolText.Text"="Resume Session" ("Boolean Text.Text")) -> ()  [unwired: 2 in, 2 out]
                n407 = property on="BtnS: Stop Session" class="Bool"("DisabledEnum"=w812, "BoolText.Text"="Stop Session" ("Boolean Text.Text")) -> ()  [unwired: 2 in, 2 out]
                n408 = property on="BtnS: Pause Session" class="Bool"("DisabledEnum"=w814, "BoolText.Text"="Paused" ("Boolean Text.Text")) -> ()  [unwired: 2 in, 2 out]
                n409 = property on="BtnSI: Inspect Session" class="Bool"("DisabledEnum"=w814, "BoolText.Text"="Stop first" ("Boolean Text.Text")) -> ()  [unwired: 2 in, 2 out]
              }
              frame "Wait for Response" {
                w822 = T17."Disabled and Grayed Out" ("Disabled")
                w820 = T17."Enabled" ("Disabled")
                n410 = property on="BtnS: Start/Resume Session" class="Bool"("Blinking"=FALSE, "DisabledEnum"=w820, "BoolText.Text"="Resume Session" ("Boolean Text.Text")) -> ()  [unwired: 2 in, 2 out]
                n411 = property on="BtnS: Stop Session" class="Bool"("DisabledEnum"=w820, "BoolText.Text"="Stop Session" ("Boolean Text.Text")) -> ()  [unwired: 2 in, 2 out]
                n412 = property on="BtnS: Pause Session" class="Bool"("DisabledEnum"=w822, "BoolText.Text"="Paused" ("Boolean Text.Text")) -> ()  [unwired: 2 in, 2 out]
                n413 = property on="BtnSI: Inspect Session" class="Bool"("DisabledEnum"=w822, "BoolText.Text"="Stop first" ("Boolean Text.Text")) -> ()  [unwired: 2 in, 2 out]
              }
              frame "Stop" {
                w824 = T17."Enabled" ("Disabled")
                n414 = property on="BtnS: Start/Resume Session" class="Bool"("Blinking"=FALSE, "DisabledEnum"=w824, "BoolText.Text"="Restart Session" ("Boolean Text.Text")) -> ()  [unwired: 2 in, 2 out]
                n415 = property on="BtnS: Stop Session" class="Bool"("DisabledEnum"=w824, "BoolText.Text"="Exit" ("Boolean Text.Text")) -> ()  [unwired: 2 in, 2 out]
                n416 = property on="BtnSI: Inspect Session" class="Bool"("DisabledEnum"=w824, "BoolText.Text"="Inspect Data" ("Boolean Text.Text")) -> ()  [unwired: 2 in, 2 out]
                n417 = property on="BtnS: Pause Session" class="Bool"("DisabledEnum"=T17."Disabled and Grayed Out" ("Disabled"), "BoolText.Text"="Not Active" ("Boolean Text.Text")) -> ()  [unwired: 2 in, 2 out]
              }
              frame "Restart" {
              }
              frame "Inspect" {
              }
              frame "Exit" {
              }
              frame "Active Session" {
              }
              frame "Wait to begin" {
              }
            }
            n418 = call "Console Entry.vi"("Error In"=w799, "Data In"=w800, "Console Entry"=w798) -> ("Data out"=w801:T6)  [unwired: 8 in]
          }
          event Timeout {
            # "Not in use"
            n419 = event-data() -> ()  [unwired: 1 in, 1 out]
          }
        }
      }
      frame Error {
        w843 = TRUE  # Shutdown Program
        # "Software shutsdown if an error is detected."
        n420 = call "Console Entry.vi"("Error In"=w839, "Data In"=w841, "Console Entry"="An error has occured in GUI-loop. GUI Software shutting down.") -> ("Data out"=w842:T6)  [unwired: 8 in]
      }
    }
    n421 = Unbundle By Name(w97) -> ("Console log"=→"GUI Console log":string, "CPU(ms)"=w92:u32)
    n422 = Unbundle By Name(w97) -> ("Result Data.Diff"=→"Diff":bool[], "Result Data.Tx Byte"=→"Tx Log":string[], "Result Data.Rx Byte"=→"Rx Log":string[], "Result Data.Send Log"=→"Send Log":string[], "Result Data.Parsed Data.Tx Running States"=→"Tx Running States":string[], "Result Data.Parsed Data.Tx Error"=→"Tx Error?":bool[], "Result Data.Parsed Data.Tx MIDI Tag"=→"Tx MIDI Message Type":string[], "Result Data.Parsed Data.Tx MIDI Parsed Data"=→"Tx Parsed Data":string[], "Result Data.Parsed Data.Diff"=→"Diff":bool[], "Result Data.Parsed Data.Rx MIDI Parsed Data"=→"Rx Parsed Data":string[], "Result Data.Parsed Data.Rx MIDI Tag"=→"Rx MIDI Message Type":string[], "Result Data.Parsed Data.Rx Error"=→"Rx Error?":bool[], "Result Data.Parsed Data.Rx Running States"=→"Rx Running States":string[])
    n423 = Wait (ms)(milliseconds to wait=w92) -> ()  [unwired: 1 out]
  }
  n424 = control-ref of="This VI"() -> (w48:refnum<vi>)
  n425 = property class="VI"(reference=w48, "Description"="The main Graphical User Interface" ("VI Description"), "TB.Visible"=w9, "Front Panel.Resizeable"=w6, "Front Panel.IsFrontmost"=w8, "Front Panel.ShowMenuBar"=w7, "Front Panel.Closeable"=w4, "Front Panel.Minimizeable"=TRUE ("Front Panel Window:Minimizable"), "Front Panel.TitleBarVis"=w3, "Front Panel.KeepWinProps"=w1, "Front Panel.Title"="MIDI Dev Tool" ("Front Panel Window:Title")) -> (reference out=w16:refnum<vi>, error out=w14:errorcluster, "Hist.Revision"=→"Revision Number":u32, "Front Panel.PanelBounds"=w18:T24)  [unwired: 1 in]
  n426 = property on="GUI Tab" class="TabCtl (strict)"("Tabs Visible?"=TRUE) -> ("Height"=w10:u32, "Width"=w13:u32)  [unwired: 2 in, 2 out]
  n427 = Unbundle By Name(w18) -> ("Top"=w22:i16, "Left"=w19:i16)
  n428 = Add(x=w22, y=w10) -> (x+y=w21:u32)
  n429 = Add(x=w19, y=w13) -> (x+y=w20:u32)
  n430 = Bundle By Name(cluster=w18, "Bottom"=w21, "Right"=w20) -> (w15:T24)
  n431 = property on="Window size" class="VI"(reference=w16, error in=w14, "Front Panel.PanelBounds"=w15) -> (reference out=w17:refnum<vi>)  [unwired: 1 out]
  n432 = property on="Pane" class="Pane"("Origin"=T14 {"Horizontal"=0, "Vertical"=0}) -> ()  [unwired: 2 in, 2 out]
  n433 = Close Reference(reference=w17) -> ()  [unwired: 1 in, 1 out]
  n434 = Current VI's Path() -> (path=w58:path)
  n435 = Strip Path(path=w58) -> (stripped path=→"VI Path":path, name=w36:string)
  "VI-filename" <- w36
  n436 = Search and Replace String(input string=w36, search string=".vi") -> (result string=→"VI-Name":string)  [unwired: 6 in, 3 out]
  n437 = control-ref of="This VI"() -> (w53:refnum<vi>)
  n438 = Number To Decimal String(number=w25) -> (decimal integer string=w26:string)  [unwired: 1 in]
  n439 = invoke on="Invoke Node" class="VI" method="FP.Close"(reference=w53, error in=w41) -> (error out=w46:errorcluster)  [unwired: 1 in, 2 out]
  "Error Out" <- w46
  n440 = Concatenate Strings("GUI closed after " ("Console Entry"), w26, " iterations.") -> (w28:string)
  n441 = call "Console Entry.vi"("Error In"=w46, "Data In"=w43, "Console Entry"=w28) -> ("Data out"=→"Data out":T6)  [unwired: 8 in]
  n442 = call <vilib>:"Simple Error Handler.vi"("type of dialog (OK msg:1)"=w40, "error in (no error)"=w41) -> ("message"=→"Error Message":string)  [unwired: 3 in, 4 out]
